vi "TestCloneAPI.vi"() -> ()   [LabVIEW 2014, in "AppModule.lvlib"]
uses:
  AppModule.lvlib
  Modules/EventPlugins/EventPluginBaseClass/TypeDefs/clEvtReportArray.ctl
  Modules/EventPlugins/EventPluginBaseClass/TypeDefs/clEvtReport.ctl
  TestInfo.ctl
  <userlib>/NIST/ModuleAdminLib/ModuleAdmin/ModuleAdmin.lvclass
  PublicAPI/Arguments/Broadcasts/clDidInit.ctl
  <userlib>/NIST/ModuleAdminLib/ModuleAdmin/ModuleAdmin.lvclass/ModuleAdmin.ctl
  PublicAPI/Arguments/Requests/clStopArgument.ctl
  PublicAPI/Arguments/Broadcasts/clStatUpdate.ctl
  PublicAPI/Arguments/Broadcasts/clErrorRpt.ctl
  <userlib>/NIST/ModuleAdminLib/ModuleAdmin/Accessors/Read CloneRegRef.vi
  <userlib>/NIST/ModuleAdminLib/CloneRegistration/CloneRegistration.lvclass
  AppPlugins/AppPluginBaseClass/AppPluginsBase.lvclass
  Modules/EventPlugins/EventPluginBaseClass/EventPluginBaseClass.lvclass
panel:
  in  "Show Panel":bool=TRUE
  in  "clEvtReportArray":T1=[{"Timestamp"=0.0, "Synx"=[568.0+0.0i, 1.190780345954324-0.33374089306165294i], "Freq"=0.0, "ROCOF"=0.0, "ID"=0}, {"Timestamp"=0.016666666666666666, "Synx"=[568.0+0.0i, 1.1810969656424384-0.32546333931377436i], "Freq"=0.0, "ROCOF"=0.0, "ID"=0}, {"Timestamp"=0.03333333333333333, "Synx"=[568.0+0.0i, 1.1693115287267182-0.31671147728228455i], "Freq"=0.0, "ROCOF"=0.0, "ID"=0}, {"Timestamp"=0.05, "Synx"=[568.0+0.0i, 1.1606529094889346-0.31107310083226175i], "Freq"=0.0, "ROCOF"=0.0, "ID"=0}, {"Timestamp"=0.06666666666666667, "Synx"=[568.0+0.0i, 1.1511600610436028-0.3062276131124402i], "Freq"=0.0, "ROCOF"=0.0, "ID"=0}, {"Timestamp"=0.08333333333333333, "Synx"=[568.0+0.0i, 1.141837461613581-0.29981509873354867i], "Freq"=0.0, "ROCOF"=0.0, "ID"=0}, {"Timestamp"=0.1, "Synx"=[568.0+0.0i, 1.132999689101532-0.29386587405402154i], "Freq"=0.0, "ROCOF"=0.0, "ID"=0}, {"Timestamp"=0.11666666666666667, "Synx"=[568.0+0.0i, 1.120988242874583-0.289722818423098i], "Freq"=0.0, "ROCOF"=0.0, "ID"=0}, {"Timestamp"=0.13333333333333333, "Synx"=[568.0+0.0i, 1.1078960385040597-0.2847668931047751i], "Freq"=0.0, "ROCOF"=0.0, "ID"=0}, {"Timestamp"=0.15, "Synx"=[568.0+0.0i, 1.096899084625727-0.27749439848438295i], "Freq"=0.0, "ROCOF"=0.0, "ID"=0}, {"Timestamp"=0.16666666666666666, "Synx"=[568.0+0.0i, 1.0850742831418392-0.27039791150864656i], "Freq"=0.0, "ROCOF"=0.0, "ID"=0}, {"Timestamp"=0.18333333333333332, "Synx"=[568.0+0.0i, 1.0713145693136845-0.2651913268468527i], "Freq"=0.0, "ROCOF"=0.0, "ID"=0}, {"Timestamp"=0.2, "Synx"=[568.0+0.0i, 1.058651026567817-0.26009080544434765i], "Freq"=0.0, "ROCOF"=0.0, "ID"=0}, {"Timestamp"=0.21666666666666667, "Synx"=[568.0+0.0i, 1.047567941555359-0.2538376451665603i], "Freq"=0.0, "ROCOF"=0.0, "ID"=0}, {"Timestamp"=0.23333333333333334, "Synx"=[568.0+0.0i, 1.0372285324721322-0.24790510395917895i], "Freq"=0.0, "ROCOF"=0.0, "ID"=0}, {"Timestamp"=0.25, "Synx"=[568.0+0.0i, 1.0281270236165359-0.24308381241327934i], "Freq"=0.0, "ROCOF"=0.0, "ID"=0}, {"Timestamp"=0.26666666666666666, "Synx"=[568.0+0.0i, 1.019518023697579-0.23787936057061518i], "Freq"=0.0, "ROCOF"=0.0, "ID"=0}, {"Timestamp"=0.2833333333333333, "Synx"=[568.0+0.0i, 1.010800255948057-0.23161401369825027i], "Freq"=0.0, "ROCOF"=0.0, "ID"=0}, {"Timestamp"=0.3, "Synx"=[568.0+0.0i, 1.003674388169744-0.22570699751690862i], "Freq"=0.0, "ROCOF"=0.0, "ID"=0}, {"Timestamp"=0.31666666666666665, "Synx"=[568.0+0.0i, 0.9986163027163525-0.2209187376418739i], "Freq"=0.0, "ROCOF"=0.0, "ID"=0}, {"Timestamp"=0.3333333333333333, "Synx"=[568.0+0.0i, 0.9938645348874-0.2162117736588246i], "Freq"=0.0, "ROCOF"=0.0, "ID"=0}, {"Timestamp"=0.35, "Synx"=[568.0+0.0i, 0.9888741952521247-0.21098043381559242i], "Freq"=0.0, "ROCOF"=0.0, "ID"=0}, {"Timestamp"=0.36666666666666664, "Synx"=[568.0+0.0i, 0.9845024487867219-0.2059636015094523i], "Freq"=0.0, "ROCOF"=0.0, "ID"=0}, {"Timestamp"=0.3833333333333333, "Synx"=[568.0+0.0i, 0.9812997021203121-0.20152897973013287i], "Freq"=0.0, "ROCOF"=0.0, "ID"=0}, {"Timestamp"=0.4, "Synx"=[568.0+0.0i, 0.9796686282331802-0.19707208766276244i], "Freq"=0.0, "ROCOF"=0.0, "ID"=0}, {"Timestamp"=0.4166666666666667, "Synx"=[568.0+0.0i, 0.9793689209737946-0.19239063538468282i], "Freq"=0.0, "ROCOF"=0.0, "ID"=0}, {"Timestamp"=0.43333333333333335, "Synx"=[568.0+0.0i, 0.9791223588762832-0.1880765496182969i], "Freq"=0.0, "ROCOF"=0.0, "ID"=0}, {"Timestamp"=0.45, "Synx"=[568.0+0.0i, 0.9784076012133255-0.1844030678057659i], "Freq"=0.0, "ROCOF"=0.0, "ID"=0}, {"Timestamp"=0.4666666666666667, "Synx"=[568.0+0.0i, 0.9780437001103851-0.18098904356917112i], "Freq"=0.0, "ROCOF"=0.0, "ID"=0}, {"Timestamp"=0.48333333333333334, "Synx"=[568.0+0.0i, 0.9785362600845192-0.17758017606549348i], "Freq"=0.0, "ROCOF"=0.0, "ID"=0}, {"Timestamp"=0.5, "Synx"=[568.0+0.0i, 0.9796244098460881-0.17433591395465478i], "Freq"=0.0, "ROCOF"=0.0, "ID"=0}, {"Timestamp"=0.5166666666666666, "Synx"=[568.0+0.0i, 0.9809907883308882-0.1714080682319968i], "Freq"=0.0, "ROCOF"=0.0, "ID"=0}, {"Timestamp"=0.5333333333333333, "Synx"=[568.0+0.0i, 0.9823274872886526-0.1687723495865902i], "Freq"=0.0, "ROCOF"=0.0, "ID"=0}, {"Timestamp"=0.55, "Synx"=[568.0+0.0i, 0.983462189784411-0.16638817596516153i], "Freq"=0.0, "ROCOF"=0.0, "ID"=0}, {"Timestamp"=0.5666666666666667, "Synx"=[568.0+0.0i, 0.9845485154103119-0.16426564040278965i], "Freq"=0.0, "ROCOF"=0.0, "ID"=0}, {"Timestamp"=0.5833333333333334, "Synx"=[568.0+0.0i, 0.985584239414064-0.16246859604208552i], "Freq"=0.0, "ROCOF"=0.0, "ID"=0}, {"Timestamp"=0.6, "Synx"=[568.0+0.0i, 0.9863346432943544-0.16105384859898314i], "Freq"=0.0, "ROCOF"=0.0, "ID"=0}, {"Timestamp"=0.6166666666666667, "Synx"=[568.0+0.0i, 0.9869274594120697-0.15990173325766183i], "Freq"=0.0, "ROCOF"=0.0, "ID"=0}, {"Timestamp"=0.6333333333333333, "Synx"=[568.0+0.0i, 0.9877478039011985-0.15881079172447463i], "Freq"=0.0, "ROCOF"=0.0, "ID"=0}, {"Timestamp"=0.65, "Synx"=[568.0+0.0i, 0.9888213981027627-0.1578654238392025i], "Freq"=0.0, "ROCOF"=0.0, "ID"=0}, {"Timestamp"=0.6666666666666666, "Synx"=[568.0+0.0i, 0.9897899903655655-0.15735170958451475i], "Freq"=0.0, "ROCOF"=0.0, "ID"=0}, {"Timestamp"=0.6833333333333333, "Synx"=[568.0+0.0i, 0.9902590603581615-0.1572358602350405i], "Freq"=0.0, "ROCOF"=0.0, "ID"=0}, {"Timestamp"=0.7, "Synx"=[568.0+0.0i, 0.9900784555069161-0.1572161214368345i], "Freq"=0.0, "ROCOF"=0.0, "ID"=0}, {"Timestamp"=0.7166666666666667, "Synx"=[568.0+0.0i, 0.9895278777753364-0.15731883208372763i], "Freq"=0.0, "ROCOF"=0.0, "ID"=0}, {"Timestamp"=0.7333333333333333, "Synx"=[568.0+0.0i, 0.989080021975212-0.15783474992005986i], "Freq"=0.0, "ROCOF"=0.0, "ID"=0}, {"Timestamp"=0.75, "Synx"=[568.0+0.0i, 0.9888954176011563-0.15867390179905863i], "Freq"=0.0, "ROCOF"=0.0, "ID"=0}, {"Timestamp"=0.7666666666666666, "Synx"=[568.0+0.0i, 0.9887907146989974-0.15947984484815012i], "Freq"=0.0, "ROCOF"=0.0, "ID"=0}, {"Timestamp"=0.7833333333333333, "Synx"=[568.0+0.0i, 0.988608996673257-0.16034377151198184i], "Freq"=0.0, "ROCOF"=0.0, "ID"=0}, {"Timestamp"=0.8, "Synx"=[568.0+0.0i, 0.9883639010187703-0.1616590571620086i], "Freq"=0.0, "ROCOF"=0.0, "ID"=0}, {"Timestamp"=0.8166666666666667, "Synx"=[568.0+0.0i, 0.9881300871093198-0.16334744819900263i], "Freq"=0.0, "ROCOF"=0.0, "ID"=0}, {"Timestamp"=0.8333333333333334, "Synx"=[568.0+0.0i, 0.987935563942819-0.16500334964923496i], "Freq"=0.0, "ROCOF"=0.0, "ID"=0}, {"Timestamp"=0.85, "Synx"=[568.0+0.0i, 0.9877272718483234-0.16667789833021487i], "Freq"=0.0, "ROCOF"=0.0, "ID"=0}, {"Timestamp"=0.8666666666666667, "Synx"=[568.0+0.0i, 0.9874788298271437-0.16872615151931622i], "Freq"=0.0, "ROCOF"=0.0, "ID"=0}, {"Timestamp"=0.8833333333333333, "Synx"=[568.0+0.0i, 0.9873308956075638-0.17104345531162607i], "Freq"=0.0, "ROCOF"=0.0, "ID"=0}, {"Timestamp"=0.9, "Synx"=[568.0+0.0i, 0.9875023373183677-0.17325359135812915i], "Freq"=0.0, "ROCOF"=0.0, "ID"=0}, {"Timestamp"=0.9166666666666666, "Synx"=[568.0+0.0i, 0.9880769375409788-0.17546082716302083i], "Freq"=0.0, "ROCOF"=0.0, "ID"=0}, {"Timestamp"=0.9333333333333333, "Synx"=[568.0+0.0i, 0.9889727901975919-0.17803061343025103i], "Freq"=0.0, "ROCOF"=0.0, "ID"=0}, {"Timestamp"=0.95, "Synx"=[568.0+0.0i, 0.9900716675954723-0.18084239270538446i], "Freq"=0.0, "ROCOF"=0.0, "ID"=0}, {"Timestamp"=0.9666666666666667, "Synx"=[568.0+0.0i, 0.9913138098801285-0.18351383569509552i], "Freq"=0.0, "ROCOF"=0.0, "ID"=0}, {"Timestamp"=0.9833333333333333, "Synx"=[568.0+0.0i, 0.9927059395134809-0.18612156281840864i], "Freq"=0.0, "ROCOF"=0.0, "ID"=0}, {"Timestamp"=1.0, "Synx"=[568.0+0.0i, 0.9942725500443967-0.1889802065654681i], "Freq"=0.0, "ROCOF"=0.0, "ID"=0}, {"Timestamp"=1.0166666666666666, "Synx"=[568.0+0.0i, 0.9960210845304401-0.1919725771479106i], "Freq"=0.0, "ROCOF"=0.0, "ID"=0}, {"Timestamp"=1.0333333333333332, "Synx"=[568.0+0.0i, 0.9979834612527839-0.19478167183195672i], "Freq"=0.0, "ROCOF"=0.0, "ID"=0}, {"Timestamp"=1.05, "Synx"=[568.0+0.0i, 1.0002484972804047-0.19751167064157604i], "Freq"=0.0, "ROCOF"=0.0, "ID"=0}, {"Timestamp"=1.0666666666666667, "Synx"=[568.0+0.0i, 1.002881503846297-0.2004414761928846i], "Freq"=0.0, "ROCOF"=0.0, "ID"=0}, {"Timestamp"=1.0833333333333333, "Synx"=[568.0+0.0i, 1.0058207005416482-0.20344096741953177i], "Freq"=0.0, "ROCOF"=0.0, "ID"=0}, {"Timestamp"=1.1, "Synx"=[568.0+0.0i, 1.0088930396474078-0.2062160694422747i], "Freq"=0.0, "ROCOF"=0.0, "ID"=0}, {"Timestamp"=1.1166666666666667, "Synx"=[568.0+0.0i, 1.0119366213904846-0.20885167018899184i], "Freq"=0.0, "ROCOF"=0.0, "ID"=0}, {"Timestamp"=1.1333333333333333, "Synx"=[568.0+0.0i, 1.0149119748644622-0.2115806058800036i], "Freq"=0.0, "ROCOF"=0.0, "ID"=0}, {"Timestamp"=1.15, "Synx"=[568.0+0.0i, 1.0179056810778668-0.21429542627327752i], "Freq"=0.0, "ROCOF"=0.0, "ID"=0}, {"Timestamp"=1.1666666666666667, "Synx"=[568.0+0.0i, 1.0210247997149353-0.21677028291320208i], "Freq"=0.0, "ROCOF"=0.0, "ID"=0}, {"Timestamp"=1.1833333333333333, "Synx"=[568.0+0.0i, 1.0242904121615224-0.21909326464360904i], "Freq"=0.0, "ROCOF"=0.0, "ID"=0}, {"Timestamp"=1.2, "Synx"=[568.0+0.0i, 1.0276294409622935-0.22144760825551188i], "Freq"=0.0, "ROCOF"=0.0, "ID"=0}, {"Timestamp"=1.2166666666666666, "Synx"=[568.0+0.0i, 1.0309366382600036-0.22372454940306044i], "Freq"=0.0, "ROCOF"=0.0, "ID"=0}, {"Timestamp"=1.2333333333333334, "Synx"=[568.0+0.0i, 1.034122599519737-0.22573253429899973i], "Freq"=0.0, "ROCOF"=0.0, "ID"=0}, {"Timestamp"=1.25, "Synx"=[568.0+0.0i, 1.0371248961434893-0.22754465011227762i], "Freq"=0.0, "ROCOF"=0.0, "ID"=0}, {"Timestamp"=1.2666666666666666, "Synx"=[568.0+0.0i, 1.0399089328448776-0.22930943033456028i], "Freq"=0.0, "ROCOF"=0.0, "ID"=0}, {"Timestamp"=1.2833333333333332, "Synx"=[568.0+0.0i, 1.0424748833879-0.23094818360098296i], "Freq"=0.0, "ROCOF"=0.0, "ID"=0}, {"Timestamp"=1.3, "Synx"=[568.0+0.0i, 1.0448588007734052-0.23232432995386262i], "Freq"=0.0, "ROCOF"=0.0, "ID"=0}, {"Timestamp"=1.3166666666666667, "Synx"=[568.0+0.0i, 1.0471046614265525-0.2334997597566502i], "Freq"=0.0, "ROCOF"=0.0, "ID"=0}, {"Timestamp"=1.3333333333333333, "Synx"=[568.0+0.0i, 1.0492147693375238-0.2345797734322047i], "Freq"=0.0, "ROCOF"=0.0, "ID"=0}, {"Timestamp"=1.35, "Synx"=[568.0+0.0i, 1.051127469782084-0.23549558631738093i], "Freq"=0.0, "ROCOF"=0.0, "ID"=0}, {"Timestamp"=1.3666666666666667, "Synx"=[568.0+0.0i, 1.0527518253261423-0.23614499855661975i], "Freq"=0.0, "ROCOF"=0.0, "ID"=0}, {"Timestamp"=1.3833333333333333, "Synx"=[568.0+0.0i, 1.0540260126145868-0.23657909568574823i], "Freq"=0.0, "ROCOF"=0.0, "ID"=0}, {"Timestamp"=1.4, "Synx"=[568.0+0.0i, 1.054945892663717-0.2368819323041705i], "Freq"=0.0, "ROCOF"=0.0, "ID"=0}, {"Timestamp"=1.4166666666666667, "Synx"=[568.0+0.0i, 1.0555482675331331-0.23701405871573272i], "Freq"=0.0, "ROCOF"=0.0, "ID"=0}, {"Timestamp"=1.4333333333333333, "Synx"=[568.0+0.0i, 1.0558754196772442-0.23691094249154757i], "Freq"=0.0, "ROCOF"=0.0, "ID"=0}, {"Timestamp"=1.45, "Synx"=[568.0+0.0i, 1.0559544563236483-0.23660818628452154i], "Freq"=0.0, "ROCOF"=0.0, "ID"=0}, {"Timestamp"=1.4666666666666666, "Synx"=[568.0+0.0i, 1.055797989100892-0.23616063145396285i], "Freq"=0.0, "ROCOF"=0.0, "ID"=0}, {"Timestamp"=1.4833333333333334, "Synx"=[568.0+0.0i, 1.055406843586187-0.23554395055091526i], "Freq"=0.0, "ROCOF"=0.0, "ID"=0}, {"Timestamp"=1.5, "Synx"=[568.0+0.0i, 1.054764636174528-0.2347207410253123i], "Freq"=0.0, "ROCOF"=0.0, "ID"=0}, {"Timestamp"=1.5166666666666666, "Synx"=[568.0+0.0i, 1.053839485044776-0.23371891599675987i], "Freq"=0.0, "ROCOF"=0.0, "ID"=0}, {"Timestamp"=1.5333333333333332, "Synx"=[568.0+0.0i, 1.052606256276664-0.23258210431801657i], "Freq"=0.0, "ROCOF"=0.0, "ID"=0}, {"Timestamp"=1.55, "Synx"=[568.0+0.0i, 1.0510755677912442-0.23130805513800712i], "Freq"=0.0, "ROCOF"=0.0, "ID"=0}, {"Timestamp"=1.5666666666666667, "Synx"=[568.0+0.0i, 1.049301705484443-0.2298801248778193i], "Freq"=0.0, "ROCOF"=0.0, "ID"=0}, {"Timestamp"=1.5833333333333333, "Synx"=[568.0+0.0i, 1.0473582415628429-0.22831163248547198i], "Freq"=0.0, "ROCOF"=0.0, "ID"=0}, {"Timestamp"=1.6, "Synx"=[568.0+0.0i, 1.045299722988945-0.2266294223502902i], "Freq"=0.0, "ROCOF"=0.0, "ID"=0}, {"Timestamp"=1.6166666666666667, "Synx"=[568.0+0.0i, 1.0431401466637653-0.22484454637484289i], "Freq"=0.0, "ROCOF"=0.0, "ID"=0}, {"Timestamp"=1.6333333333333333, "Synx"=[568.0+0.0i, 1.040861588268909-0.22295697150093405i], "Freq"=0.0, "ROCOF"=0.0, "ID"=0}, {"Timestamp"=1.65, "Synx"=[568.0+0.0i, 1.0384399620313718-0.22097421707535697i], "Freq"=0.0, "ROCOF"=0.0, "ID"=0}, {"Timestamp"=1.6666666666666667, "Synx"=[568.0+0.0i, 1.0358675042297611-0.21891745552321926i], "Freq"=0.0, "ROCOF"=0.0, "ID"=0}, {"Timestamp"=1.6833333333333333, "Synx"=[568.0+0.0i, 1.0331629251005825-0.21681001277654294i], "Freq"=0.0, "ROCOF"=0.0, "ID"=0}, {"Timestamp"=1.7, "Synx"=[568.0+0.0i, 1.0303703614372581-0.2146595394080782i], "Freq"=0.0, "ROCOF"=0.0, "ID"=0}, {"Timestamp"=1.7166666666666666, "Synx"=[568.0+0.0i, 1.0275489835542104-0.21246241961811713i], "Freq"=0.0, "ROCOF"=0.0, "ID"=0}, {"Timestamp"=1.7333333333333334, "Synx"=[568.0+0.0i, 1.0247542957426232-0.2102314718081312i], "Freq"=0.0, "ROCOF"=0.0, "ID"=0}, {"Timestamp"=1.75, "Synx"=[568.0+0.0i, 1.0220173416906368-0.20799789534335755i], "Freq"=0.0, "ROCOF"=0.0, "ID"=0}, {"Timestamp"=1.7666666666666666, "Synx"=[568.0+0.0i, 1.0193349786964445-0.2057764748395524i], "Freq"=0.0, "ROCOF"=0.0, "ID"=0}, {"Timestamp"=1.7833333333333332, "Synx"=[568.0+0.0i, 1.0166813461179105-0.20355939974713314i], "Freq"=0.0, "ROCOF"=0.0, "ID"=0}, {"Timestamp"=1.8, "Synx"=[568.0+0.0i, 1.0140349586059054-0.2013562244167269i], "Freq"=0.0, "ROCOF"=0.0, "ID"=0}, {"Timestamp"=1.8166666666666667, "Synx"=[568.0+0.0i, 1.011401946309843-0.199201567979025i], "Freq"=0.0, "ROCOF"=0.0, "ID"=0}, {"Timestamp"=1.8333333333333333, "Synx"=[568.0+0.0i, 1.0088189657709958-0.19710976685721138i], "Freq"=0.0, "ROCOF"=0.0, "ID"=0}, {"Timestamp"=1.8499999999999999, "Synx"=[568.0+0.0i, 1.0063360973300026-0.19506592883055504i], "Freq"=0.0, "ROCOF"=0.0, "ID"=0}, {"Timestamp"=1.8666666666666667, "Synx"=[568.0+0.0i, 1.0039941235484178-0.19307571606837412i], "Freq"=0.0, "ROCOF"=0.0, "ID"=0}, {"Timestamp"=1.8833333333333333, "Synx"=[568.0+0.0i, 1.0018108504340801-0.19117557136705798i], "Freq"=0.0, "ROCOF"=0.0, "ID"=0}, {"Timestamp"=1.9, "Synx"=[568.0+0.0i, 0.9997811138555077-0.1893803254456488i], "Freq"=0.0, "ROCOF"=0.0, "ID"=0}, {"Timestamp"=1.9166666666666667, "Synx"=[568.0+0.0i, 0.9978862013971358-0.18767229377489536i], "Freq"=0.0, "ROCOF"=0.0, "ID"=0}, {"Timestamp"=1.9333333333333333, "Synx"=[568.0+0.0i, 0.9961067328730887-0.1860544329617271i], "Freq"=0.0, "ROCOF"=0.0, "ID"=0}, {"Timestamp"=1.95, "Synx"=[568.0+0.0i, 0.9944347806515849-0.18456035273097823i], "Freq"=0.0, "ROCOF"=0.0, "ID"=0}, {"Timestamp"=1.9666666666666666, "Synx"=[568.0+0.0i, 0.9928809871930054-0.183200624078482i], "Freq"=0.0, "ROCOF"=0.0, "ID"=0}, {"Timestamp"=1.9833333333333334, "Synx"=[568.0+0.0i, 0.991472195404676-0.18195400575743148i], "Freq"=0.0, "ROCOF"=0.0, "ID"=0}, {"Timestamp"=2.0, "Synx"=[568.0+0.0i, 0.9902390140964307-0.18082137861780578i], "Freq"=0.0, "ROCOF"=0.0, "ID"=0}, {"Timestamp"=2.0166666666666666, "Synx"=[568.0+0.0i, 0.9891998068808097-0.17983365869239556i], "Freq"=0.0, "ROCOF"=0.0, "ID"=0}, {"Timestamp"=2.033333333333333, "Synx"=[568.0+0.0i, 0.9883513468000275-0.17899859462260528i], "Freq"=0.0, "ROCOF"=0.0, "ID"=0}, {"Timestamp"=2.05, "Synx"=[568.0+0.0i, 0.9876722603689594-0.1782935810602652i], "Freq"=0.0, "ROCOF"=0.0, "ID"=0}, {"Timestamp"=2.0666666666666664, "Synx"=[568.0+0.0i, 0.9871363571572059-0.17771691091941522i], "Freq"=0.0, "ROCOF"=0.0, "ID"=0}, {"Timestamp"=2.0833333333333335, "Synx"=[568.0+0.0i, 0.9867267773227768-0.1772936545888048i], "Freq"=0.0, "ROCOF"=0.0, "ID"=0}, {"Timestamp"=2.1, "Synx"=[568.0+0.0i, 0.9864430423534721-0.1770267626387451i], "Freq"=0.0, "ROCOF"=0.0, "ID"=0}, {"Timestamp"=2.1166666666666667, "Synx"=[568.0+0.0i, 0.986298827687823-0.17689282953983645i], "Freq"=0.0, "ROCOF"=0.0, "ID"=0}, {"Timestamp"=2.1333333333333333, "Synx"=[568.0+0.0i, 0.9863131477619512-0.1768887579439425i], "Freq"=0.0, "ROCOF"=0.0, "ID"=0}, {"Timestamp"=2.15, "Synx"=[568.0+0.0i, 0.9864994558429381-0.177034793451872i], "Freq"=0.0, "ROCOF"=0.0, "ID"=0}, {"Timestamp"=2.1666666666666665, "Synx"=[568.0+0.0i, 0.9868572194198217-0.1773304474284138i], "Freq"=0.0, "ROCOF"=0.0, "ID"=0}, {"Timestamp"=2.183333333333333, "Synx"=[568.0+0.0i, 0.9873699279289171-0.17775230993232238i], "Freq"=0.0, "ROCOF"=0.0, "ID"=0}, {"Timestamp"=2.2, "Synx"=[568.0+0.0i, 0.9880113409407102-0.17829500158520384i], "Freq"=0.0, "ROCOF"=0.0, "ID"=0}, {"Timestamp"=2.216666666666667, "Synx"=[568.0+0.0i, 0.9887574643840766-0.17897253600781066i], "Freq"=0.0, "ROCOF"=0.0, "ID"=0}, {"Timestamp"=2.2333333333333334, "Synx"=[568.0+0.0i, 0.9895975289188882-0.1797808520503357i], "Freq"=0.0, "ROCOF"=0.0, "ID"=0}, {"Timestamp"=2.25, "Synx"=[568.0+0.0i, 0.9905370349611532-0.18069754891558917i], "Freq"=0.0, "ROCOF"=0.0, "ID"=0}, {"Timestamp"=2.2666666666666666, "Synx"=[568.0+0.0i, 0.9915908737833355-0.18171619390982416i], "Freq"=0.0, "ROCOF"=0.0, "ID"=0}, {"Timestamp"=2.283333333333333, "Synx"=[568.0+0.0i, 0.9927710926045651-0.18284584848506485i], "Freq"=0.0, "ROCOF"=0.0, "ID"=0}, {"Timestamp"=2.3, "Synx"=[568.0+0.0i, 0.9940769861581061-0.18407991133459486i], "Freq"=0.0, "ROCOF"=0.0, "ID"=0}, {"Timestamp"=2.3166666666666664, "Synx"=[568.0+0.0i, 0.9954929513614348-0.18539704332928741i], "Freq"=0.0, "ROCOF"=0.0, "ID"=0}, {"Timestamp"=2.3333333333333335, "Synx"=[568.0+0.0i, 0.9969943464528188-0.1867891587045225i], "Freq"=0.0, "ROCOF"=0.0, "ID"=0}, {"Timestamp"=2.35, "Synx"=[568.0+0.0i, 0.9985573425247952-0.1882603465051167i], "Freq"=0.0, "ROCOF"=0.0, "ID"=0}, {"Timestamp"=2.3666666666666667, "Synx"=[568.0+0.0i, 1.000167483038519-0.1898022846290975i], "Freq"=0.0, "ROCOF"=0.0, "ID"=0}, {"Timestamp"=2.3833333333333333, "Synx"=[568.0+0.0i, 1.0018229554400828-0.1913957013938104i], "Freq"=0.0, "ROCOF"=0.0, "ID"=0}, {"Timestamp"=2.4, "Synx"=[568.0+0.0i, 1.0035312090473962-0.193031959160047i], "Freq"=0.0, "ROCOF"=0.0, "ID"=0}, {"Timestamp"=2.4166666666666665, "Synx"=[568.0+0.0i, 1.0053006517591185-0.19471146411512794i], "Freq"=0.0, "ROCOF"=0.0, "ID"=0}, {"Timestamp"=2.433333333333333, "Synx"=[568.0+0.0i, 1.0071317484332953-0.1964249403531514i], "Freq"=0.0, "ROCOF"=0.0, "ID"=0}, {"Timestamp"=2.45, "Synx"=[568.0+0.0i, 1.0090124582136468-0.19815504239043605i], "Freq"=0.0, "ROCOF"=0.0, "ID"=0}, {"Timestamp"=2.466666666666667, "Synx"=[568.0+0.0i, 1.0109206703555722-0.19989252092690646i], "Freq"=0.0, "ROCOF"=0.0, "ID"=0}, {"Timestamp"=2.4833333333333334, "Synx"=[568.0+0.0i, 1.0128321538239238-0.20163494496273376i], "Freq"=0.0, "ROCOF"=0.0, "ID"=0}, {"Timestamp"=2.5, "Synx"=[568.0+0.0i, 1.0147292338719154-0.20337322647478442i], "Freq"=0.0, "ROCOF"=0.0, "ID"=0}, {"Timestamp"=2.5166666666666666, "Synx"=[568.0+0.0i, 1.0166052330789968-0.20509277039788493i], "Freq"=0.0, "ROCOF"=0.0, "ID"=0}, {"Timestamp"=2.533333333333333, "Synx"=[568.0+0.0i, 1.018462594764228-0.2067846555469391i], "Freq"=0.0, "ROCOF"=0.0, "ID"=0}, {"Timestamp"=2.55, "Synx"=[568.0+0.0i, 1.0203063349318222-0.2084447732784657i], "Freq"=0.0, "ROCOF"=0.0, "ID"=0}, {"Timestamp"=2.5666666666666664, "Synx"=[568.0+0.0i, 1.0221366959972835-0.21006478864608596i], "Freq"=0.0, "ROCOF"=0.0, "ID"=0}, {"Timestamp"=2.5833333333333335, "Synx"=[568.0+0.0i, 1.0239447597183418-0.21163276568005002i], "Freq"=0.0, "ROCOF"=0.0, "ID"=0}, {"Timestamp"=2.6, "Synx"=[568.0+0.0i, 1.0257129589008291-0.21314046586550892i], "Freq"=0.0, "ROCOF"=0.0, "ID"=0}, {"Timestamp"=2.6166666666666667, "Synx"=[568.0+0.0i, 1.027420017866818-0.21458324661005146i], "Freq"=0.0, "ROCOF"=0.0, "ID"=0}, {"Timestamp"=2.6333333333333333, "Synx"=[568.0+0.0i, 1.0290477789233554-0.21595454514215445i], "Freq"=0.0, "ROCOF"=0.0, "ID"=0}, {"Timestamp"=2.65, "Synx"=[568.0+0.0i, 1.0305864073218247-0.21724562789289598i], "Freq"=0.0, "ROCOF"=0.0, "ID"=0}, {"Timestamp"=2.6666666666666665, "Synx"=[568.0+0.0i, 1.0320352004463418-0.21844964155200813i], "Freq"=0.0, "ROCOF"=0.0, "ID"=0}, {"Timestamp"=2.683333333333333, "Synx"=[568.0+0.0i, 1.033398558605959-0.21956228647542675i], "Freq"=0.0, "ROCOF"=0.0, "ID"=0}, {"Timestamp"=2.7, "Synx"=[568.0+0.0i, 1.0346794259610796-0.220579103490274i], "Freq"=0.0, "ROCOF"=0.0, "ID"=0}, {"Timestamp"=2.716666666666667, "Synx"=[568.0+0.0i, 1.0358739695934602-0.22149449595483597i], "Freq"=0.0, "ROCOF"=0.0, "ID"=0}, {"Timestamp"=2.7333333333333334, "Synx"=[568.0+0.0i, 1.0369704525709336-0.22230344771707009i], "Freq"=0.0, "ROCOF"=0.0, "ID"=0}, {"Timestamp"=2.75, "Synx"=[568.0+0.0i, 1.037952730864153-0.22300295686017155i], "Freq"=0.0, "ROCOF"=0.0, "ID"=0}, {"Timestamp"=2.7666666666666666, "Synx"=[568.0+0.0i, 1.0388062152341506-0.22359127274266685i], "Freq"=0.0, "ROCOF"=0.0, "ID"=0}, {"Timestamp"=2.783333333333333, "Synx"=[568.0+0.0i, 1.0395229873649514-0.22406610431184215i], "Freq"=0.0, "ROCOF"=0.0, "ID"=0}, {"Timestamp"=2.8, "Synx"=[568.0+0.0i, 1.0401034718302804-0.22442460907944128i], "Freq"=0.0, "ROCOF"=0.0, "ID"=0}, {"Timestamp"=2.8166666666666664, "Synx"=[568.0+0.0i, 1.0405540106953015-0.2246655131641988i], "Freq"=0.0, "ROCOF"=0.0, "ID"=0}, {"Timestamp"=2.8333333333333335, "Synx"=[568.0+0.0i, 1.040881788358684-0.22478976692268932i], "Freq"=0.0, "ROCOF"=0.0, "ID"=0}, {"Timestamp"=2.85, "Synx"=[568.0+0.0i, 1.0410898451192874-0.22479817513687864i], "Freq"=0.0, "ROCOF"=0.0, "ID"=0}, {"Timestamp"=2.8666666666666667, "Synx"=[568.0+0.0i, 1.0411748272008872-0.22469027892540053i], "Freq"=0.0, "ROCOF"=0.0, "ID"=0}, {"Timestamp"=2.8833333333333333, "Synx"=[568.0+0.0i, 1.0411286539854963-0.2244669659399703i], "Freq"=0.0, "ROCOF"=0.0, "ID"=0}, {"Timestamp"=2.9, "Synx"=[568.0+0.0i, 1.0409431383184042-0.2241319236944976i], "Freq"=0.0, "ROCOF"=0.0, "ID"=0}, {"Timestamp"=2.9166666666666665, "Synx"=[568.0+0.0i, 1.0406149486083935-0.223688776483113i], "Freq"=0.0, "ROCOF"=0.0, "ID"=0}, {"Timestamp"=2.933333333333333, "Synx"=[568.0+0.0i, 1.0401481469543568-0.22313931511734783i], "Freq"=0.0, "ROCOF"=0.0, "ID"=0}, {"Timestamp"=2.95, "Synx"=[568.0+0.0i, 1.0395529880638208-0.22248648096840987i], "Freq"=0.0, "ROCOF"=0.0, "ID"=0}, {"Timestamp"=2.966666666666667, "Synx"=[568.0+0.0i, 1.0388418160687836-0.22173628896227382i], "Freq"=0.0, "ROCOF"=0.0, "ID"=0}, {"Timestamp"=2.9833333333333334, "Synx"=[568.0+0.0i, 1.038024445035296-0.22089469991740576i], "Freq"=0.0, "ROCOF"=0.0, "ID"=0}, {"Timestamp"=3.0, "Synx"=[568.0+0.0i, 1.0371055193036594-0.21996554495909618i], "Freq"=0.0, "ROCOF"=0.0, "ID"=0}, {"Timestamp"=3.0166666666666666, "Synx"=[568.0+0.0i, 1.0360851111409897-0.21895365241069248i], "Freq"=0.0, "ROCOF"=0.0, "ID"=0}, {"Timestamp"=3.033333333333333, "Synx"=[568.0+0.0i, 1.0349620308096652-0.21786687915385072i], "Freq"=0.0, "ROCOF"=0.0, "ID"=0}, {"Timestamp"=3.05, "Synx"=[568.0+0.0i, 1.0337379556267012-0.21671286730600722i], "Freq"=0.0, "ROCOF"=0.0, "ID"=0}, {"Timestamp"=3.0666666666666664, "Synx"=[568.0+0.0i, 1.032420159355366-0.21549694207410314i], "Freq"=0.0, "ROCOF"=0.0, "ID"=0}, {"Timestamp"=3.0833333333333335, "Synx"=[568.0+0.0i, 1.0310214330160141-0.21422527222805923i], "Freq"=0.0, "ROCOF"=0.0, "ID"=0}, {"Timestamp"=3.1, "Synx"=[568.0+0.0i, 1.0295573001613536-0.21290685068428078i], "Freq"=0.0, "ROCOF"=0.0, "ID"=0}, {"Timestamp"=3.1166666666666667, "Synx"=[568.0+0.0i, 1.0280420678045863-0.21155030329001417i], "Freq"=0.0, "ROCOF"=0.0, "ID"=0}, {"Timestamp"=3.1333333333333333, "Synx"=[568.0+0.0i, 1.026485849307144-0.21016190288057138i], "Freq"=0.0, "ROCOF"=0.0, "ID"=0}, {"Timestamp"=3.15, "Synx"=[568.0+0.0i, 1.0248941098278908-0.20874858319455356i], "Freq"=0.0, "ROCOF"=0.0, "ID"=0}, {"Timestamp"=3.1666666666666665, "Synx"=[568.0+0.0i, 1.0232698513994773-0.20731971500730859i], "Freq"=0.0, "ROCOF"=0.0, "ID"=0}, {"Timestamp"=3.183333333333333, "Synx"=[568.0+0.0i, 1.0216171056391063-0.20588410095269838i], "Freq"=0.0, "ROCOF"=0.0, "ID"=0}, {"Timestamp"=3.2, "Synx"=[568.0+0.0i, 1.019943757010864-0.2044482358246055i], "Freq"=0.0, "ROCOF"=0.0, "ID"=0}, {"Timestamp"=3.216666666666667, "Synx"=[568.0+0.0i, 1.0182621888817098-0.2030191018882827i], "Freq"=0.0, "ROCOF"=0.0, "ID"=0}, {"Timestamp"=3.2333333333333334, "Synx"=[568.0+0.0i, 1.0165874904108576-0.2016056949152871i], "Freq"=0.0, "ROCOF"=0.0, "ID"=0}, {"Timestamp"=3.25, "Synx"=[568.0+0.0i, 1.0149342620899795-0.20021629454728956i], "Freq"=0.0, "ROCOF"=0.0, "ID"=0}, {"Timestamp"=3.2666666666666666, "Synx"=[568.0+0.0i, 1.0133137368991374-0.19885698972394428i], "Freq"=0.0, "ROCOF"=0.0, "ID"=0}, {"Timestamp"=3.283333333333333, "Synx"=[568.0+0.0i, 1.0117326922007803-0.19753415568661703i], "Freq"=0.0, "ROCOF"=0.0, "ID"=0}, {"Timestamp"=3.3, "Synx"=[568.0+0.0i, 1.0101946352320756-0.1962557062861227i], "Freq"=0.0, "ROCOF"=0.0, "ID"=0}, {"Timestamp"=3.3166666666666664, "Synx"=[568.0+0.0i, 1.0087025314481806-0.1950287202110056i], "Freq"=0.0, "ROCOF"=0.0, "ID"=0}, {"Timestamp"=3.3333333333333335, "Synx"=[568.0+0.0i, 1.0072615430318437-0.19385826181023505i], "Freq"=0.0, "ROCOF"=0.0, "ID"=0}, {"Timestamp"=3.35, "Synx"=[568.0+0.0i, 1.005880279054299-0.19274951304727636i], "Freq"=0.0, "ROCOF"=0.0, "ID"=0}, {"Timestamp"=3.3666666666666667, "Synx"=[568.0+0.0i, 1.0045699077788675-0.19170876632512351i], "Freq"=0.0, "ROCOF"=0.0, "ID"=0}, {"Timestamp"=3.3833333333333333, "Synx"=[568.0+0.0i, 1.003341668412867-0.19074142641550254i], "Freq"=0.0, "ROCOF"=0.0, "ID"=0}, {"Timestamp"=3.4, "Synx"=[568.0+0.0i, 1.0022041752236373-0.1898510876973532i], "Freq"=0.0, "ROCOF"=0.0, "ID"=0}, {"Timestamp"=3.4166666666666665, "Synx"=[568.0+0.0i, 1.0011619643035912-0.18904129443643466i], "Freq"=0.0, "ROCOF"=0.0, "ID"=0}, {"Timestamp"=3.433333333333333, "Synx"=[568.0+0.0i, 1.0002159963486787-0.1883163110222497i], "Freq"=0.0, "ROCOF"=0.0, "ID"=0}, {"Timestamp"=3.4499999999999997, "Synx"=[568.0+0.0i, 0.9993657447576055-0.18767952143268934i], "Freq"=0.0, "ROCOF"=0.0, "ID"=0}, {"Timestamp"=3.466666666666667, "Synx"=[568.0+0.0i, 0.9986116726251671-0.18713274128551685i], "Freq"=0.0, "ROCOF"=0.0, "ID"=0}, {"Timestamp"=3.4833333333333334, "Synx"=[568.0+0.0i, 0.9979567561916559-0.18667761728176166i], "Freq"=0.0, "ROCOF"=0.0, "ID"=0}, {"Timestamp"=3.5, "Synx"=[568.0+0.0i, 0.997406281290491-0.1863162092713793i], "Freq"=0.0, "ROCOF"=0.0, "ID"=0}, {"Timestamp"=3.5166666666666666, "Synx"=[568.0+0.0i, 0.9969660891386926-0.18604975936115342i], "Freq"=0.0, "ROCOF"=0.0, "ID"=0}, {"Timestamp"=3.533333333333333, "Synx"=[568.0+0.0i, 0.9966402670447526-0.18587818594586064i], "Freq"=0.0, "ROCOF"=0.0, "ID"=0}, {"Timestamp"=3.55, "Synx"=[568.0+0.0i, 0.9964295424714044-0.18580114488753546i], "Freq"=0.0, "ROCOF"=0.0, "ID"=0}, {"Timestamp"=3.5666666666666664, "Synx"=[568.0+0.0i, 0.9963312203782239-0.185818473874469i], "Freq"=0.0, "ROCOF"=0.0, "ID"=0}, {"Timestamp"=3.5833333333333335, "Synx"=[568.0+0.0i, 0.9963406449134696-0.18592930964841095i], "Freq"=0.0, "ROCOF"=0.0, "ID"=0}, {"Timestamp"=3.6, "Synx"=[568.0+0.0i, 0.9964533451459586-0.18613172626604754i], "Freq"=0.0, "ROCOF"=0.0, "ID"=0}, {"Timestamp"=3.6166666666666667, "Synx"=[568.0+0.0i, 0.9966666891072367-0.18642349180843512i], "Freq"=0.0, "ROCOF"=0.0, "ID"=0}, {"Timestamp"=3.6333333333333333, "Synx"=[568.0+0.0i, 0.9969801872409653-0.18680240689624547i], "Freq"=0.0, "ROCOF"=0.0, "ID"=0}, {"Timestamp"=3.65, "Synx"=[568.0+0.0i, 0.9973943537224486-0.18726571901813266i], "Freq"=0.0, "ROCOF"=0.0, "ID"=0}, {"Timestamp"=3.6666666666666665, "Synx"=[568.0+0.0i, 0.9979088128423509-0.18780986160987279i], "Freq"=0.0, "ROCOF"=0.0, "ID"=0}, {"Timestamp"=3.683333333333333, "Synx"=[568.0+0.0i, 0.9985207085784669-0.18843095232817975i], "Freq"=0.0, "ROCOF"=0.0, "ID"=0}, {"Timestamp"=3.6999999999999997, "Synx"=[568.0+0.0i, 0.9992242646278583-0.1891250659624096i], "Freq"=0.0, "ROCOF"=0.0, "ID"=0}, {"Timestamp"=3.716666666666667, "Synx"=[568.0+0.0i, 1.0000116934124799-0.18988790243732154i], "Freq"=0.0, "ROCOF"=0.0, "ID"=0}, {"Timestamp"=3.7333333333333334, "Synx"=[568.0+0.0i, 1.0008749290986005-0.19071459337633773i], "Freq"=0.0, "ROCOF"=0.0, "ID"=0}, {"Timestamp"=3.75, "Synx"=[568.0+0.0i, 1.0018072441448587-0.1915999838259529i], "Freq"=0.0, "ROCOF"=0.0, "ID"=0}, {"Timestamp"=3.7666666666666666, "Synx"=[568.0+0.0i, 1.0028039076667605-0.1925388599034244i], "Freq"=0.0, "ROCOF"=0.0, "ID"=0}, {"Timestamp"=3.783333333333333, "Synx"=[568.0+0.0i, 1.003861587242621-0.19352581616107542i], "Freq"=0.0, "ROCOF"=0.0, "ID"=0}, {"Timestamp"=3.8, "Synx"=[568.0+0.0i, 1.0049768802801915-0.19455510318750538i], "Freq"=0.0, "ROCOF"=0.0, "ID"=0}, {"Timestamp"=3.8166666666666664, "Synx"=[568.0+0.0i, 1.0061448146314809-0.19562074210389557i], "Freq"=0.0, "ROCOF"=0.0, "ID"=0}, {"Timestamp"=3.8333333333333335, "Synx"=[568.0+0.0i, 1.007358142859756-0.1967167298637634i], "Freq"=0.0, "ROCOF"=0.0, "ID"=0}, {"Timestamp"=3.85, "Synx"=[568.0+0.0i, 1.00860779497357-0.19783705895208065i], "Freq"=0.0, "ROCOF"=0.0, "ID"=0}, {"Timestamp"=3.8666666666666667, "Synx"=[568.0+0.0i, 1.0098842169175037-0.19897558468448356i], "Freq"=0.0, "ROCOF"=0.0, "ID"=0}, {"Timestamp"=3.8833333333333333, "Synx"=[568.0+0.0i, 1.011178858818969-0.20012601108108485i], "Freq"=0.0, "ROCOF"=0.0, "ID"=0}, {"Timestamp"=3.9, "Synx"=[568.0+0.0i, 1.0124850289927154-0.20128208217084906i], "Freq"=0.0, "ROCOF"=0.0, "ID"=0}, {"Timestamp"=3.9166666666666665, "Synx"=[568.0+0.0i, 1.0137977026271638-0.2024377084594979i], "Freq"=0.0, "ROCOF"=0.0, "ID"=0}, {"Timestamp"=3.933333333333333, "Synx"=[568.0+0.0i, 1.0151124491394243-0.20358684260411145i], "Freq"=0.0, "ROCOF"=0.0, "ID"=0}, {"Timestamp"=3.9499999999999997, "Synx"=[568.0+0.0i, 1.0164241049721945-0.20472337713513603i], "Freq"=0.0, "ROCOF"=0.0, "ID"=0}, {"Timestamp"=3.966666666666667, "Synx"=[568.0+0.0i, 1.0177259288041245-0.205841329585249i], "Freq"=0.0, "ROCOF"=0.0, "ID"=0}, {"Timestamp"=3.9833333333333334, "Synx"=[568.0+0.0i, 1.0190096893671852-0.2069350364625256i], "Freq"=0.0, "ROCOF"=0.0, "ID"=0}, {"Timestamp"=4.0, "Synx"=[568.0+0.0i, 1.0202666194943035-0.20799902742409807i], "Freq"=0.0, "ROCOF"=0.0, "ID"=0}, {"Timestamp"=4.016666666666667, "Synx"=[568.0+0.0i, 1.021488707710869-0.20902786387932934i], "Freq"=0.0, "ROCOF"=0.0, "ID"=0}, {"Timestamp"=4.033333333333333, "Synx"=[568.0+0.0i, 1.0226696370562114-0.21001631794052444i], "Freq"=0.0, "ROCOF"=0.0, "ID"=0}, {"Timestamp"=4.05, "Synx"=[568.0+0.0i, 1.023804896655799-0.2109596019987795i], "Freq"=0.0, "ROCOF"=0.0, "ID"=0}, {"Timestamp"=4.066666666666666, "Synx"=[568.0+0.0i, 1.024891054591562-0.21185323977060794i], "Freq"=0.0, "ROCOF"=0.0, "ID"=0}, {"Timestamp"=4.083333333333333, "Synx"=[568.0+0.0i, 1.0259246310194525-0.2126928728625221i], "Freq"=0.0, "ROCOF"=0.0, "ID"=0}, {"Timestamp"=4.1, "Synx"=[568.0+0.0i, 1.0269012057368159-0.21347443219995235i], "Freq"=0.0, "ROCOF"=0.0, "ID"=0}, {"Timestamp"=4.116666666666666, "Synx"=[568.0+0.0i, 1.027815240693725-0.21419437644345046i], "Freq"=0.0, "ROCOF"=0.0, "ID"=0}, {"Timestamp"=4.133333333333333, "Synx"=[568.0+0.0i, 1.0286606936923244-0.21484955774275472i], "Freq"=0.0, "ROCOF"=0.0, "ID"=0}, {"Timestamp"=4.15, "Synx"=[568.0+0.0i, 1.0294320724175916-0.2154370143219451i], "Freq"=0.0, "ROCOF"=0.0, "ID"=0}, {"Timestamp"=4.166666666666667, "Synx"=[568.0+0.0i, 1.0301253567065425-0.21595413077151254i], "Freq"=0.0, "ROCOF"=0.0, "ID"=0}, {"Timestamp"=4.183333333333334, "Synx"=[568.0+0.0i, 1.030738310204174-0.21639886717395307i], "Freq"=0.0, "ROCOF"=0.0, "ID"=0}, {"Timestamp"=4.2, "Synx"=[568.0+0.0i, 1.0312700473211396-0.2167696224841078i], "Freq"=0.0, "ROCOF"=0.0, "ID"=0}, {"Timestamp"=4.216666666666667, "Synx"=[568.0+0.0i, 1.0317201238690874-0.21706502780097908i], "Freq"=0.0, "ROCOF"=0.0, "ID"=0}, {"Timestamp"=4.233333333333333, "Synx"=[568.0+0.0i, 1.0320876628160311-0.21728409112310762i], "Freq"=0.0, "ROCOF"=0.0, "ID"=0}, {"Timestamp"=4.25, "Synx"=[568.0+0.0i, 1.0323709862346906-0.2174264030755045i], "Freq"=0.0, "ROCOF"=0.0, "ID"=0}, {"Timestamp"=4.266666666666667, "Synx"=[568.0+0.0i, 1.0325679330832016-0.2174919997093849i], "Freq"=0.0, "ROCOF"=0.0, "ID"=0}, {"Timestamp"=4.283333333333333, "Synx"=[568.0+0.0i, 1.0326766662033717-0.2174811655541134i], "Freq"=0.0, "ROCOF"=0.0, "ID"=0}, {"Timestamp"=4.3, "Synx"=[568.0+0.0i, 1.032696516494469-0.21739455963329707i], "Freq"=0.0, "ROCOF"=0.0, "ID"=0}, {"Timestamp"=4.316666666666666, "Synx"=[568.0+0.0i, 1.032628409902785-0.21723339101287625i], "Freq"=0.0, "ROCOF"=0.0, "ID"=0}, {"Timestamp"=4.333333333333333, "Synx"=[568.0+0.0i, 1.0324746641150886-0.2169992851653377i], "Freq"=0.0, "ROCOF"=0.0, "ID"=0}, {"Timestamp"=4.35, "Synx"=[568.0+0.0i, 1.0322382867936144-0.21669410280284668i], "Freq"=0.0, "ROCOF"=0.0, "ID"=0}, {"Timestamp"=4.366666666666666, "Synx"=[568.0+0.0i, 1.0319221668510608-0.21632004405306698i], "Freq"=0.0, "ROCOF"=0.0, "ID"=0}, {"Timestamp"=4.383333333333333, "Synx"=[568.0+0.0i, 1.0315285897927267-0.21587978996140247i], "Freq"=0.0, "ROCOF"=0.0, "ID"=0}, {"Timestamp"=4.4, "Synx"=[568.0+0.0i, 1.031059315962401-0.21537637559723927i], "Freq"=0.0, "ROCOF"=0.0, "ID"=0}, {"Timestamp"=4.416666666666667, "Synx"=[568.0+0.0i, 1.0305161487793255-0.21481302811973807i], "Freq"=0.0, "ROCOF"=0.0, "ID"=0}, {"Timestamp"=4.433333333333334, "Synx"=[568.0+0.0i, 1.0299016598775008-0.21419324858157454i], "Freq"=0.0, "ROCOF"=0.0, "ID"=0}, {"Timestamp"=4.45, "Synx"=[568.0+0.0i, 1.029219666363022-0.2135209204612558i], "Freq"=0.0, "ROCOF"=0.0, "ID"=0}, {"Timestamp"=4.466666666666667, "Synx"=[568.0+0.0i, 1.0284752032510356-0.212800193207802i], "Freq"=0.0, "ROCOF"=0.0, "ID"=0}, {"Timestamp"=4.483333333333333, "Synx"=[568.0+0.0i, 1.0276740139011808-0.21203534086222092i], "Freq"=0.0, "ROCOF"=0.0, "ID"=0}, {"Timestamp"=4.5, "Synx"=[568.0+0.0i, 1.0268218377851666-0.21123082152003722i], "Freq"=0.0, "ROCOF"=0.0, "ID"=0}, {"Timestamp"=4.516666666666667, "Synx"=[568.0+0.0i, 1.0259238714142305-0.21039135567697023i], "Freq"=0.0, "ROCOF"=0.0, "ID"=0}, {"Timestamp"=4.533333333333333, "Synx"=[568.0+0.0i, 1.0249846693590385-0.20952182320869708i], "Freq"=0.0, "ROCOF"=0.0, "ID"=0}, {"Timestamp"=4.55, "Synx"=[568.0+0.0i, 1.0240085048941572-0.20862714319845982i], "Freq"=0.0, "ROCOF"=0.0, "ID"=0}, {"Timestamp"=4.566666666666666, "Synx"=[568.0+0.0i, 1.0229999623391008-0.20771231341341118i], "Freq"=0.0, "ROCOF"=0.0, "ID"=0}, {"Timestamp"=4.583333333333333, "Synx"=[568.0+0.0i, 1.0219644181800682-0.20678246365890895i], "Freq"=0.0, "ROCOF"=0.0, "ID"=0}, {"Timestamp"=4.6, "Synx"=[568.0+0.0i, 1.0209081414341832-0.20584276862808254i], "Freq"=0.0, "ROCOF"=0.0, "ID"=0}, {"Timestamp"=4.616666666666666, "Synx"=[568.0+0.0i, 1.019837958287597-0.2048983482948202i], "Freq"=0.0, "ROCOF"=0.0, "ID"=0}, {"Timestamp"=4.633333333333333, "Synx"=[568.0+0.0i, 1.0187606612577174-0.2039542901482685i], "Freq"=0.0, "ROCOF"=0.0, "ID"=0}, {"Timestamp"=4.65, "Synx"=[568.0+0.0i, 1.0176824724470745-0.20301568323249433i], "Freq"=0.0, "ROCOF"=0.0, "ID"=0}, {"Timestamp"=4.666666666666667, "Synx"=[568.0+0.0i, 1.0166088290059523-0.20208754869715048i], "Freq"=0.0, "ROCOF"=0.0, "ID"=0}, {"Timestamp"=4.683333333333334, "Synx"=[568.0+0.0i, 1.0155445757016979-0.20117476017908312i], "Freq"=0.0, "ROCOF"=0.0, "ID"=0}, {"Timestamp"=4.7, "Synx"=[568.0+0.0i, 1.0144944282605235-0.2002820527688007i], "Freq"=0.0, "ROCOF"=0.0, "ID"=0}, {"Timestamp"=4.716666666666667, "Synx"=[568.0+0.0i, 1.0134634319864066-0.1994140437502579i], "Freq"=0.0, "ROCOF"=0.0, "ID"=0}, {"Timestamp"=4.733333333333333, "Synx"=[568.0+0.0i, 1.0124571543964993-0.19857518159877913i], "Freq"=0.0, "ROCOF"=0.0, "ID"=0}, {"Timestamp"=4.75, "Synx"=[568.0+0.0i, 1.011481504371806-0.19776968495819794i], "Freq"=0.0, "ROCOF"=0.0, "ID"=0}, {"Timestamp"=4.766666666666667, "Synx"=[568.0+0.0i, 1.0105422754123117-0.19700154216335072i], "Freq"=0.0, "ROCOF"=0.0, "ID"=0}, {"Timestamp"=4.783333333333333, "Synx"=[568.0+0.0i, 1.0096446549572584-0.19627452418880523i], "Freq"=0.0, "ROCOF"=0.0, "ID"=0}, {"Timestamp"=4.8, "Synx"=[568.0+0.0i, 1.0087929506207438-0.19559215223284185i], "Freq"=0.0, "ROCOF"=0.0, "ID"=0}, {"Timestamp"=4.816666666666666, "Synx"=[568.0+0.0i, 1.0079906585542548-0.19495765400981588i], "Freq"=0.0, "ROCOF"=0.0, "ID"=0}, {"Timestamp"=4.833333333333333, "Synx"=[568.0+0.0i, 1.0072408118301963-0.19437395771311453i], "Freq"=0.0, "ROCOF"=0.0, "ID"=0}, {"Timestamp"=4.85, "Synx"=[568.0+0.0i, 1.006546400456679-0.19384370174687732i], "Freq"=0.0, "ROCOF"=0.0, "ID"=0}, {"Timestamp"=4.866666666666666, "Synx"=[568.0+0.0i, 1.005910625874371-0.1933692198843506i], "Freq"=0.0, "ROCOF"=0.0, "ID"=0}, {"Timestamp"=4.883333333333333, "Synx"=[568.0+0.0i, 1.0053368521044037-0.19295251302975772i], "Freq"=0.0, "ROCOF"=0.0, "ID"=0}, {"Timestamp"=4.9, "Synx"=[568.0+0.0i, 1.004828284781337-0.19259524087171695i], "Freq"=0.0, "ROCOF"=0.0, "ID"=0}, {"Timestamp"=4.916666666666667, "Synx"=[568.0+0.0i, 1.0043875548199743-0.1922987319555496i], "Freq"=0.0, "ROCOF"=0.0, "ID"=0}, {"Timestamp"=4.933333333333334, "Synx"=[568.0+0.0i, 1.0040164284605368-0.19206398487620052i], "Freq"=0.0, "ROCOF"=0.0, "ID"=0}, {"Timestamp"=4.95, "Synx"=[568.0+0.0i, 1.003715789864982-0.1918916536401944i], "Freq"=0.0, "ROCOF"=0.0, "ID"=0}, {"Timestamp"=4.966666666666667, "Synx"=[568.0+0.0i, 1.0034858916720504-0.19178203958029608i], "Freq"=0.0, "ROCOF"=0.0, "ID"=0}, {"Timestamp"=4.983333333333333, "Synx"=[568.0+0.0i, 1.0033267267960733-0.19173510396979637i], "Freq"=0.0, "ROCOF"=0.0, "ID"=0}, {"Timestamp"=5.0, "Synx"=[568.0+0.0i, 1.0032383170353087-0.1917504828516047i], "Freq"=0.0, "ROCOF"=0.0, "ID"=0}, {"Timestamp"=5.016666666666667, "Synx"=[568.0+0.0i, 1.0032207681445935-0.19182748378399625i], "Freq"=0.0, "ROCOF"=0.0, "ID"=0}, {"Timestamp"=5.033333333333333, "Synx"=[568.0+0.0i, 1.0032740733264955-0.19196507978054253i], "Freq"=0.0, "ROCOF"=0.0, "ID"=0}, {"Timestamp"=5.05, "Synx"=[568.0+0.0i, 1.0033977835652619-0.19216192565092038i], "Freq"=0.0, "ROCOF"=0.0, "ID"=0}, {"Timestamp"=5.066666666666666, "Synx"=[568.0+0.0i, 1.003590730686606-0.19241638377355708i], "Freq"=0.0, "ROCOF"=0.0, "ID"=0}, {"Timestamp"=5.083333333333333, "Synx"=[568.0+0.0i, 1.0038509542236131-0.19272652994260053i], "Freq"=0.0, "ROCOF"=0.0, "ID"=0}, {"Timestamp"=5.1, "Synx"=[568.0+0.0i, 1.004175868899983-0.19309015022434953i], "Freq"=0.0, "ROCOF"=0.0, "ID"=0}, {"Timestamp"=5.116666666666666, "Synx"=[568.0+0.0i, 1.0045625801768623-0.19350476106002978i], "Freq"=0.0, "ROCOF"=0.0, "ID"=0}, {"Timestamp"=5.133333333333333, "Synx"=[568.0+0.0i, 1.0050081806979294-0.19396764290124094i], "Freq"=0.0, "ROCOF"=0.0, "ID"=0}, {"Timestamp"=5.15, "Synx"=[568.0+0.0i, 1.0055098783389436-0.19447585277475907i], "Freq"=0.0, "ROCOF"=0.0, "ID"=0}, {"Timestamp"=5.166666666666667, "Synx"=[568.0+0.0i, 1.0060649036030218-0.19502622427673633i], "Freq"=0.0, "ROCOF"=0.0, "ID"=0}, {"Timestamp"=5.183333333333334, "Synx"=[568.0+0.0i, 1.0066702651055675-0.19561539078837775i], "Freq"=0.0, "ROCOF"=0.0, "ID"=0}, {"Timestamp"=5.2, "Synx"=[568.0+0.0i, 1.0073225010639546-0.19623982390795303i], "Freq"=0.0, "ROCOF"=0.0, "ID"=0}, {"Timestamp"=5.216666666666667, "Synx"=[568.0+0.0i, 1.0080175713529735-0.1968958503668058i], "Freq"=0.0, "ROCOF"=0.0, "ID"=0}, {"Timestamp"=5.233333333333333, "Synx"=[568.0+0.0i, 1.008750954000322-0.19757965469950775i], "Freq"=0.0, "ROCOF"=0.0, "ID"=0}, {"Timestamp"=5.25, "Synx"=[568.0+0.0i, 1.009517898369839-0.19828730426648097i], "Freq"=0.0, "ROCOF"=0.0, "ID"=0}, {"Timestamp"=5.266666666666667, "Synx"=[568.0+0.0i, 1.0103137057438232-0.19901478947683637i], "Freq"=0.0, "ROCOF"=0.0, "ID"=0}, {"Timestamp"=5.283333333333333, "Synx"=[568.0+0.0i, 1.0111338989628946-0.19975804281680093i], "Freq"=0.0, "ROCOF"=0.0, "ID"=0}, {"Timestamp"=5.3, "Synx"=[568.0+0.0i, 1.011974208068996-0.20051294335999878i], "Freq"=0.0, "ROCOF"=0.0, "ID"=0}, {"Timestamp"=5.316666666666666, "Synx"=[568.0+0.0i, 1.0128304005333102-0.20127534203383415i], "Freq"=0.0, "ROCOF"=0.0, "ID"=0}, {"Timestamp"=5.333333333333333, "Synx"=[568.0+0.0i, 1.0136980667561373-0.20204110090717126i], "Freq"=0.0, "ROCOF"=0.0, "ID"=0}, {"Timestamp"=5.35, "Synx"=[568.0+0.0i, 1.0145724909533393-0.2028061122437551i], "Freq"=0.0, "ROCOF"=0.0, "ID"=0}, {"Timestamp"=5.366666666666666, "Synx"=[568.0+0.0i, 1.0154486864516232-0.20356630367786796i], "Freq"=0.0, "ROCOF"=0.0, "ID"=0}, {"Timestamp"=5.383333333333333, "Synx"=[568.0+0.0i, 1.0163215830353902-0.20431766200395626i], "Freq"=0.0, "ROCOF"=0.0, "ID"=0}, {"Timestamp"=5.4, "Synx"=[568.0+0.0i, 1.017186272897865-0.20505626917260925i], "Freq"=0.0, "ROCOF"=0.0, "ID"=0}, {"Timestamp"=5.416666666666667, "Synx"=[568.0+0.0i, 1.0180381939513956-0.20577831957778667i], "Freq"=0.0, "ROCOF"=0.0, "ID"=0}, {"Timestamp"=5.433333333333334, "Synx"=[568.0+0.0i, 1.0188731674461204-0.2064801246645199i], "Freq"=0.0, "ROCOF"=0.0, "ID"=0}, {"Timestamp"=5.45, "Synx"=[568.0+0.0i, 1.019687287870982-0.20715813362910207i], "Freq"=0.0, "ROCOF"=0.0, "ID"=0}, {"Timestamp"=5.466666666666667, "Synx"=[568.0+0.0i, 1.0204767418285008-0.20780896421385514i], "Freq"=0.0, "ROCOF"=0.0, "ID"=0}, {"Timestamp"=5.483333333333333, "Synx"=[568.0+0.0i, 1.0212376669482748-0.20842941671823828i], "Freq"=0.0, "ROCOF"=0.0, "ID"=0}, {"Timestamp"=5.5, "Synx"=[568.0+0.0i, 1.0219661353679779-0.2090164768094309i], "Freq"=0.0, "ROCOF"=0.0, "ID"=0}, {"Timestamp"=5.516666666666667, "Synx"=[568.0+0.0i, 1.022658275575987-0.20956733173869277i], "Freq"=0.0, "ROCOF"=0.0, "ID"=0}, {"Timestamp"=5.533333333333333, "Synx"=[568.0+0.0i, 1.0233104711490006-0.21007939455433494i], "Freq"=0.0, "ROCOF"=0.0, "ID"=0}, {"Timestamp"=5.55, "Synx"=[568.0+0.0i, 1.0239195355971182-0.21055031373185776i], "Freq"=0.0, "ROCOF"=0.0, "ID"=0}, {"Timestamp"=5.566666666666666, "Synx"=[568.0+0.0i, 1.024482778726415-0.21097797316322878i], "Freq"=0.0, "ROCOF"=0.0, "ID"=0}, {"Timestamp"=5.583333333333333, "Synx"=[568.0+0.0i, 1.0249979407111536-0.2113605028517062i], "Freq"=0.0, "ROCOF"=0.0, "ID"=0}, {"Timestamp"=5.6, "Synx"=[568.0+0.0i, 1.0254630410800945-0.2116962956869903i], "Freq"=0.0, "ROCOF"=0.0, "ID"=0}, {"Timestamp"=5.616666666666666, "Synx"=[568.0+0.0i, 1.0258762326320552-0.2119840119736437i], "Freq"=0.0, "ROCOF"=0.0, "ID"=0}, {"Timestamp"=5.633333333333333, "Synx"=[568.0+0.0i, 1.0262357431408762-0.2122225758454484i], "Freq"=0.0, "ROCOF"=0.0, "ID"=0}, {"Timestamp"=5.65, "Synx"=[568.0+0.0i, 1.0265399364697667-0.21241117984147273i], "Freq"=0.0, "ROCOF"=0.0, "ID"=0}, {"Timestamp"=5.666666666666667, "Synx"=[568.0+0.0i, 1.0267874586350758-0.21254929396092387i], "Freq"=0.0, "ROCOF"=0.0, "ID"=0}, {"Timestamp"=5.683333333333334, "Synx"=[568.0+0.0i, 1.0269773894303111-0.2126366648296583i], "Freq"=0.0, "ROCOF"=0.0, "ID"=0}, {"Timestamp"=5.7, "Synx"=[568.0+0.0i, 1.0271093196300742-0.21267330816440977i], "Freq"=0.0, "ROCOF"=0.0, "ID"=0}, {"Timestamp"=5.716666666666667, "Synx"=[568.0+0.0i, 1.0271833160397073-0.21265950710959472i], "Freq"=0.0, "ROCOF"=0.0, "ID"=0}, {"Timestamp"=5.733333333333333, "Synx"=[568.0+0.0i, 1.0271997973722957-0.21259581381102438i], "Freq"=0.0, "ROCOF"=0.0, "ID"=0}, {"Timestamp"=5.75, "Synx"=[568.0+0.0i, 1.0271593898685838-0.21248304339029167i], "Freq"=0.0, "ROCOF"=0.0, "ID"=0}, {"Timestamp"=5.766666666666667, "Synx"=[568.0+0.0i, 1.0270628387511458-0.2123222624951767i], "Freq"=0.0, "ROCOF"=0.0, "ID"=0}, {"Timestamp"=5.783333333333333, "Synx"=[568.0+0.0i, 1.0269110177718923-0.2121147817793899i], "Freq"=0.0, "ROCOF"=0.0, "ID"=0}, {"Timestamp"=5.8, "Synx"=[568.0+0.0i, 1.0267050240640663-0.21186215074935488i], "Freq"=0.0, "ROCOF"=0.0, "ID"=0}, {"Timestamp"=5.816666666666666, "Synx"=[568.0+0.0i, 1.0264462995872217-0.2115661471530367i], "Freq"=0.0, "ROCOF"=0.0, "ID"=0}, {"Timestamp"=5.833333333333333, "Synx"=[568.0+0.0i, 1.0261367078722872-0.2112287620722902i], "Freq"=0.0, "ROCOF"=0.0, "ID"=0}, {"Timestamp"=5.85, "Synx"=[568.0+0.0i, 1.0257785209086585-0.2108521873778944i], "Freq"=0.0, "ROCOF"=0.0, "ID"=0}, {"Timestamp"=5.866666666666666, "Synx"=[568.0+0.0i, 1.0253743202915657-0.21043880502271173i], "Freq"=0.0, "ROCOF"=0.0, "ID"=0}, {"Timestamp"=5.883333333333333, "Synx"=[568.0+0.0i, 1.0249268618384257-0.20999117282257618i], "Freq"=0.0, "ROCOF"=0.0, "ID"=0}, {"Timestamp"=5.9, "Synx"=[568.0+0.0i, 1.0244389698227974-0.20951200693322497i], "Freq"=0.0, "ROCOF"=0.0, "ID"=0}, {"Timestamp"=5.916666666666667, "Synx"=[568.0+0.0i, 1.0239135078543238-0.20900416551069814i], "Freq"=0.0, "ROCOF"=0.0, "ID"=0}, {"Timestamp"=5.933333333333334, "Synx"=[568.0+0.0i, 1.0233534299718436-0.20847063396657708i], "Freq"=0.0, "ROCOF"=0.0, "ID"=0}, {"Timestamp"=5.95, "Synx"=[568.0+0.0i, 1.0227618719809528-0.2079145084163386i], "Freq"=0.0, "ROCOF"=0.0, "ID"=0}, {"Timestamp"=5.966666666666667, "Synx"=[568.0+0.0i, 1.022142222765238-0.20733897668418672i], "Freq"=0.0, "ROCOF"=0.0, "ID"=0}, {"Timestamp"=5.983333333333333, "Synx"=[568.0+0.0i, 1.021498128147648-0.20674729967071157i], "Freq"=0.0, "ROCOF"=0.0, "ID"=0}, {"Timestamp"=6.0, "Synx"=[568.0+0.0i, 1.0208334176405367-0.20614279429029359i], "Freq"=0.0, "ROCOF"=0.0, "ID"=0}, {"Timestamp"=6.016666666666667, "Synx"=[568.0+0.0i, 1.0201519858666082-0.20552881604780754i], "Freq"=0.0, "ROCOF"=0.0, "ID"=0}, {"Timestamp"=6.033333333333333, "Synx"=[568.0+0.0i, 1.0194576832234792-0.20490873991398156i], "Freq"=0.0, "ROCOF"=0.0, "ID"=0}, {"Timestamp"=6.05, "Synx"=[568.0+0.0i, 1.0187542630660906-0.20428594105425504i], "Freq"=0.0, "ROCOF"=0.0, "ID"=0}, {"Timestamp"=6.066666666666666, "Synx"=[568.0+0.0i, 1.0180454004335766-0.20366377724140172i], "Freq"=0.0, "ROCOF"=0.0, "ID"=0}, {"Timestamp"=6.083333333333333, "Synx"=[568.0+0.0i, 1.0173347584360033-0.20304557207577323i], "Freq"=0.0, "ROCOF"=0.0, "ID"=0}, {"Timestamp"=6.1, "Synx"=[568.0+0.0i, 1.0166260539450658-0.2024345971290324i], "Freq"=0.0, "ROCOF"=0.0, "ID"=0}, {"Timestamp"=6.116666666666666, "Synx"=[568.0+0.0i, 1.0159230767086482-0.20183405367997492i], "Freq"=0.0, "ROCOF"=0.0, "ID"=0}, {"Timestamp"=6.133333333333333, "Synx"=[568.0+0.0i, 1.0152296430001035-0.20124705631630044i], "Freq"=0.0, "ROCOF"=0.0, "ID"=0}, {"Timestamp"=6.15, "Synx"=[568.0+0.0i, 1.014549500963457-0.20067661823495747i], "Freq"=0.0, "ROCOF"=0.0, "ID"=0}, {"Timestamp"=6.166666666666667, "Synx"=[568.0+0.0i, 1.0138862302545553-0.20012563597621974i], "Freq"=0.0, "ROCOF"=0.0, "ID"=0}, {"Timestamp"=6.183333333333334, "Synx"=[568.0+0.0i, 1.0132431802218138-0.19959687366545237i], "Freq"=0.0, "ROCOF"=0.0, "ID"=0}, {"Timestamp"=6.2, "Synx"=[568.0+0.0i, 1.0126234688123772-0.1990929493019679i], "Freq"=0.0, "ROCOF"=0.0, "ID"=0}, {"Timestamp"=6.216666666666667, "Synx"=[568.0+0.0i, 1.0120300314064534-0.19861632336292911i], "Freq"=0.0, "ROCOF"=0.0, "ID"=0}, {"Timestamp"=6.233333333333333, "Synx"=[568.0+0.0i, 1.0114656829748736-0.1981692872344395i], "Freq"=0.0, "ROCOF"=0.0, "ID"=0}, {"Timestamp"=6.25, "Synx"=[568.0+0.0i, 1.0109331518407374-0.197753951176059i], "Freq"=0.0, "ROCOF"=0.0, "ID"=0}, {"Timestamp"=6.266666666666667, "Synx"=[568.0+0.0i, 1.0104350607923511-0.19737223446232027i], "Freq"=0.0, "ROCOF"=0.0, "ID"=0}, {"Timestamp"=6.283333333333333, "Synx"=[568.0+0.0i, 1.0099738610631097-0.19702585819835639i], "Freq"=0.0, "ROCOF"=0.0, "ID"=0}, {"Timestamp"=6.3, "Synx"=[568.0+0.0i, 1.009551750320851-0.19671633823888654i], "Freq"=0.0, "ROCOF"=0.0, "ID"=0}, {"Timestamp"=6.316666666666666, "Synx"=[568.0+0.0i, 1.0091706137414975-0.19644497771432234i], "Freq"=0.0, "ROCOF"=0.0, "ID"=0}, {"Timestamp"=6.333333333333333, "Synx"=[568.0+0.0i, 1.0088320139546334-0.19621286177352854i], "Freq"=0.0, "ROCOF"=0.0, "ID"=0}, {"Timestamp"=6.35, "Synx"=[568.0+0.0i, 1.0085372291212298-0.19602085512474196i], "Freq"=0.0, "ROCOF"=0.0, "ID"=0}, {"Timestamp"=6.366666666666666, "Synx"=[568.0+0.0i, 1.0082873133758927-0.1958695998416328i], "Freq"=0.0, "ROCOF"=0.0, "ID"=0}, {"Timestamp"=6.383333333333333, "Synx"=[568.0+0.0i, 1.0080831436699635-0.19575951285176574i], "Freq"=0.0, "ROCOF"=0.0, "ID"=0}, {"Timestamp"=6.4, "Synx"=[568.0+0.0i, 1.0079254265332382-0.19569078557318276i], "Freq"=0.0, "ROCOF"=0.0, "ID"=0}, {"Timestamp"=6.416666666666667, "Synx"=[568.0+0.0i, 1.0078146615445531-0.19566338627014904i], "Freq"=0.0, "ROCOF"=0.0, "ID"=0}, {"Timestamp"=6.433333333333334, "Synx"=[568.0+0.0i, 1.0077510823377387-0.19567706272792604i], "Freq"=0.0, "ROCOF"=0.0, "ID"=0}, {"Timestamp"=6.45, "Synx"=[568.0+0.0i, 1.007734607867396-0.19573134465210343i], "Freq"=0.0, "ROCOF"=0.0, "ID"=0}, {"Timestamp"=6.466666666666667, "Synx"=[568.0+0.0i, 1.0077648305431648-0.19582554803494076i], "Freq"=0.0, "ROCOF"=0.0, "ID"=0}, {"Timestamp"=6.483333333333333, "Synx"=[568.0+0.0i, 1.007841047719826-0.19595878199615868i], "Freq"=0.0, "ROCOF"=0.0, "ID"=0}, {"Timestamp"=6.5, "Synx"=[568.0+0.0i, 1.0079623202454662-0.19612995590227128i], "Freq"=0.0, "ROCOF"=0.0, "ID"=0}, {"Timestamp"=6.516666666666667, "Synx"=[568.0+0.0i, 1.0081275286239941-0.19633778620261616i], "Freq"=0.0, "ROCOF"=0.0, "ID"=0}, {"Timestamp"=6.533333333333333, "Synx"=[568.0+0.0i, 1.008335400480432-0.19658080495036076i], "Freq"=0.0, "ROCOF"=0.0, "ID"=0}, {"Timestamp"=6.55, "Synx"=[568.0+0.0i, 1.0085845000801428-0.19685737042886595i], "Freq"=0.0, "ROCOF"=0.0, "ID"=0}, {"Timestamp"=6.566666666666666, "Synx"=[568.0+0.0i, 1.0088731919381742-0.19716567793859616i], "Freq"=0.0, "ROCOF"=0.0, "ID"=0}, {"Timestamp"=6.583333333333333, "Synx"=[568.0+0.0i, 1.0091996044918439-0.19750377023750895i], "Freq"=0.0, "ROCOF"=0.0, "ID"=0}, {"Timestamp"=6.6, "Synx"=[568.0+0.0i, 1.0095616192366983-0.19786954930479192i], "Freq"=0.0, "ROCOF"=0.0, "ID"=0}, {"Timestamp"=6.616666666666666, "Synx"=[568.0+0.0i, 1.0099568965423726-0.19826078975988917i], "Freq"=0.0, "ROCOF"=0.0, "ID"=0}, {"Timestamp"=6.633333333333333, "Synx"=[568.0+0.0i, 1.0103829297191271-0.19867515226897692i], "Freq"=0.0, "ROCOF"=0.0, "ID"=0}, {"Timestamp"=6.6499999999999995, "Synx"=[568.0+0.0i, 1.0108371045363154-0.19911019649379813i], "Freq"=0.0, "ROCOF"=0.0, "ID"=0}, {"Timestamp"=6.666666666666667, "Synx"=[568.0+0.0i, 1.0113167397747398-0.19956339495147388i], "Freq"=0.0, "ROCOF"=0.0, "ID"=0}, {"Timestamp"=6.683333333333334, "Synx"=[568.0+0.0i, 1.0118190958684263-0.200032148040241i], "Freq"=0.0, "ROCOF"=0.0, "ID"=0}, {"Timestamp"=6.7, "Synx"=[568.0+0.0i, 1.0123413565780426-0.20051379884758816i], "Freq"=0.0, "ROCOF"=0.0, "ID"=0}, {"Timestamp"=6.716666666666667, "Synx"=[568.0+0.0i, 1.0128806030991186-0.20100564735605836i], "Freq"=0.0, "ROCOF"=0.0, "ID"=0}, {"Timestamp"=6.733333333333333, "Synx"=[568.0+0.0i, 1.0134338034419772-0.2015049651288832i], "Freq"=0.0, "ROCOF"=0.0, "ID"=0}, {"Timestamp"=6.75, "Synx"=[568.0+0.0i, 1.0139978309401765-0.20200901067223118i], "Freq"=0.0, "ROCOF"=0.0, "ID"=0}, {"Timestamp"=6.766666666666667, "Synx"=[568.0+0.0i, 1.0145695096662446-0.20251504436753046i], "Freq"=0.0, "ROCOF"=0.0, "ID"=0}, {"Timestamp"=6.783333333333333, "Synx"=[568.0+0.0i, 1.0151456702554698-0.20302034264290236i], "Freq"=0.0, "ROCOF"=0.0, "ID"=0}, {"Timestamp"=6.8, "Synx"=[568.0+0.0i, 1.0157231947302792-0.20352221220606537i], "Freq"=0.0, "ROCOF"=0.0, "ID"=0}, {"Timestamp"=6.816666666666666, "Synx"=[568.0+0.0i, 1.016299035623175-0.20401800449800253i], "Freq"=0.0, "ROCOF"=0.0, "ID"=0}, {"Timestamp"=6.833333333333333, "Synx"=[568.0+0.0i, 1.0168702089504078-0.20450512951948177i], "Freq"=0.0, "ROCOF"=0.0, "ID"=0}, {"Timestamp"=6.85, "Synx"=[568.0+0.0i, 1.0174337744527369-0.2049810687452471i], "Freq"=0.0, "ROCOF"=0.0, "ID"=0}, {"Timestamp"=6.866666666666666, "Synx"=[568.0+0.0i, 1.0179868225893536-0.20544338772306536i], "Freq"=0.0, "ROCOF"=0.0, "ID"=0}, {"Timestamp"=6.883333333333333, "Synx"=[568.0+0.0i, 1.0185264831182472-0.20588974849898417i], "Freq"=0.0, "ROCOF"=0.0, "ID"=0}, {"Timestamp"=6.8999999999999995, "Synx"=[568.0+0.0i, 1.019049957652842-0.20631792125343554i], "Freq"=0.0, "ROCOF"=0.0, "ID"=0}, {"Timestamp"=6.916666666666667, "Synx"=[568.0+0.0i, 1.0195545653330853-0.20672579490079968i], "Freq"=0.0, "ROCOF"=0.0, "ID"=0}, {"Timestamp"=6.933333333333334, "Synx"=[568.0+0.0i, 1.0200377838183203-0.20711138706245194i], "Freq"=0.0, "ROCOF"=0.0, "ID"=0}, {"Timestamp"=6.95, "Synx"=[568.0+0.0i, 1.0204972706526574-0.20747285355282002i], "Freq"=0.0, "ROCOF"=0.0, "ID"=0}, {"Timestamp"=6.966666666666667, "Synx"=[568.0+0.0i, 1.0209308607508083-0.20780849696516712i], "Freq"=0.0, "ROCOF"=0.0, "ID"=0}, {"Timestamp"=6.983333333333333, "Synx"=[568.0+0.0i, 1.0213365482576342-0.2081167741410059i], "Freq"=0.0, "ROCOF"=0.0, "ID"=0}, {"Timestamp"=7.0, "Synx"=[568.0+0.0i, 1.0217124685822259-0.20839630278447058i], "Freq"=0.0, "ROCOF"=0.0, "ID"=0}, {"Timestamp"=7.016666666666667, "Synx"=[568.0+0.0i, 1.0220568951629048-0.2086458673709673i], "Freq"=0.0, "ROCOF"=0.0, "ID"=0}, {"Timestamp"=7.033333333333333, "Synx"=[568.0+0.0i, 1.0223682565126408-0.20886442410634623i], "Freq"=0.0, "ROCOF"=0.0, "ID"=0}, {"Timestamp"=7.05, "Synx"=[568.0+0.0i, 1.0226451674678076-0.20905110474672664i], "Freq"=0.0, "ROCOF"=0.0, "ID"=0}, {"Timestamp"=7.066666666666666, "Synx"=[568.0+0.0i, 1.0228864606512666-0.20920521942769854i], "Freq"=0.0, "ROCOF"=0.0, "ID"=0}, {"Timestamp"=7.083333333333333, "Synx"=[568.0+0.0i, 1.023091204049602-0.20932625866889984i], "Freq"=0.0, "ROCOF"=0.0, "ID"=0}, {"Timestamp"=7.1, "Synx"=[568.0+0.0i, 1.0232586980367784-0.20941389444740505i], "Freq"=0.0, "ROCOF"=0.0, "ID"=0}, {"Timestamp"=7.116666666666666, "Synx"=[568.0+0.0i, 1.0233884558677107-0.2094679801728417i], "Freq"=0.0, "ROCOF"=0.0, "ID"=0}, {"Timestamp"=7.133333333333333, "Synx"=[568.0+0.0i, 1.0234801797616884-0.20948854963237526i], "Freq"=0.0, "ROCOF"=0.0, "ID"=0}, {"Timestamp"=7.1499999999999995, "Synx"=[568.0+0.0i, 1.0235337459725793-0.20947581509052987i], "Freq"=0.0, "ROCOF"=0.0, "ID"=0}, {"Timestamp"=7.166666666666667, "Synx"=[568.0+0.0i, 1.0235492062993437-0.20943016454356364i], "Freq"=0.0, "ROCOF"=0.0, "ID"=0}, {"Timestamp"=7.183333333333334, "Synx"=[568.0+0.0i, 1.0235268038072345-0.20935215798166698i], "Freq"=0.0, "ROCOF"=0.0, "ID"=0}, {"Timestamp"=7.2, "Synx"=[568.0+0.0i, 1.0234669924469897-0.20924252267332918i], "Freq"=0.0, "ROCOF"=0.0, "ID"=0}, {"Timestamp"=7.216666666666667, "Synx"=[568.0+0.0i, 1.0233704480406158-0.20910214767424257i], "Freq"=0.0, "ROCOF"=0.0, "ID"=0}, {"Timestamp"=7.233333333333333, "Synx"=[568.0+0.0i, 1.023238062698138-0.2089320776384665i], "Freq"=0.0, "ROCOF"=0.0, "ID"=0}, {"Timestamp"=7.25, "Synx"=[568.0+0.0i, 1.0230709234030493-0.2087335058036809i], "Freq"=0.0, "ROCOF"=0.0, "ID"=0}, {"Timestamp"=7.266666666666667, "Synx"=[568.0+0.0i, 1.0228702834475891-0.2085077661321164i], "Freq"=0.0, "ROCOF"=0.0, "ID"=0}, {"Timestamp"=7.283333333333333, "Synx"=[568.0+0.0i, 1.0226375383925943-0.20825632482218i], "Freq"=0.0, "ROCOF"=0.0, "ID"=0}, {"Timestamp"=7.3, "Synx"=[568.0+0.0i, 1.0223742148731905-0.20798077132126996i], "Freq"=0.0, "ROCOF"=0.0, "ID"=0}, {"Timestamp"=7.316666666666666, "Synx"=[568.0+0.0i, 1.022081972928589-0.207682808728459i], "Freq"=0.0, "ROCOF"=0.0, "ID"=0}, {"Timestamp"=7.333333333333333, "Synx"=[568.0+0.0i, 1.0217626148709067-0.2073642435512425i], "Freq"=0.0, "ROCOF"=0.0, "ID"=0}, {"Timestamp"=7.35, "Synx"=[568.0+0.0i, 1.02141809012921-0.20702697503714948i], "Freq"=0.0, "ROCOF"=0.0, "ID"=0}, {"Timestamp"=7.366666666666666, "Synx"=[568.0+0.0i, 1.021050487760791-0.20667298424169578i], "Freq"=0.0, "ROCOF"=0.0, "ID"=0}, {"Timestamp"=7.383333333333333, "Synx"=[568.0+0.0i, 1.020662014966747-0.20630432273626415i], "Freq"=0.0, "ROCOF"=0.0, "ID"=0}, {"Timestamp"=7.3999999999999995, "Synx"=[568.0+0.0i, 1.020254967247349-0.20592310091279858i], "Freq"=0.0, "ROCOF"=0.0, "ID"=0}, {"Timestamp"=7.416666666666667, "Synx"=[568.0+0.0i, 1.0198316998517845-0.20553147610372663i], "Freq"=0.0, "ROCOF"=0.0, "ID"=0}, {"Timestamp"=7.433333333333334, "Synx"=[568.0+0.0i, 1.0193946089004187-0.20513164069125295i], "Freq"=0.0, "ROCOF"=0.0, "ID"=0}, {"Timestamp"=7.45, "Synx"=[568.0+0.0i, 1.0189461248868128-0.20472581012215707i], "Freq"=0.0, "ROCOF"=0.0, "ID"=0}, {"Timestamp"=7.466666666666667, "Synx"=[568.0+0.0i, 1.0184887144176185-0.20431621078332038i], "Freq"=0.0, "ROCOF"=0.0, "ID"=0}, {"Timestamp"=7.483333333333333, "Synx"=[568.0+0.0i, 1.0180248817361954-0.20390506794556904i], "Freq"=0.0, "ROCOF"=0.0, "ID"=0}, {"Timestamp"=7.5, "Synx"=[568.0+0.0i, 1.0175571620047195-0.20349459394780237i], "Freq"=0.0, "ROCOF"=0.0, "ID"=0}, {"Timestamp"=7.516666666666667, "Synx"=[568.0+0.0i, 1.017088103065574-0.2030869765473051i], "Freq"=0.0, "ROCOF"=0.0, "ID"=0}, {"Timestamp"=7.533333333333333, "Synx"=[568.0+0.0i, 1.0166202387479188-0.20268436739192922i], "Freq"=0.0, "ROCOF"=0.0, "ID"=0}, {"Timestamp"=7.55, "Synx"=[568.0+0.0i, 1.0161560612667675-0.20228887080294777i], "Freq"=0.0, "ROCOF"=0.0, "ID"=0}, {"Timestamp"=7.566666666666666, "Synx"=[568.0+0.0i, 1.0156980005563139-0.20190253302690087i], "Freq"=0.0, "ROCOF"=0.0, "ID"=0}, {"Timestamp"=7.583333333333333, "Synx"=[568.0+0.0i, 1.0152484144997211-0.2015273318891014i], "Freq"=0.0, "ROCOF"=0.0, "ID"=0}, {"Timestamp"=7.6, "Synx"=[568.0+0.0i, 1.014809588210829-0.20116516680468788i], "Freq"=0.0, "ROCOF"=0.0, "ID"=0}, {"Timestamp"=7.616666666666666, "Synx"=[568.0+0.0i, 1.0143837359753984-0.20081784931051289i], "Freq"=0.0, "ROCOF"=0.0, "ID"=0}, {"Timestamp"=7.633333333333333, "Synx"=[568.0+0.0i, 1.013972998552009-0.20048709425429811i], "Freq"=0.0, "ROCOF"=0.0, "ID"=0}, {"Timestamp"=7.6499999999999995, "Synx"=[568.0+0.0i, 1.01357943160046-0.20017451157753166i], "Freq"=0.0, "ROCOF"=0.0, "ID"=0}, {"Timestamp"=7.666666666666667, "Synx"=[568.0+0.0i, 1.0132049862415702-0.19988159864654345i], "Freq"=0.0, "ROCOF"=0.0, "ID"=0}, {"Timestamp"=7.683333333333334, "Synx"=[568.0+0.0i, 1.0128514872628045-0.1996097332645629i], "Freq"=0.0, "ROCOF"=0.0, "ID"=0}, {"Timestamp"=7.7, "Synx"=[568.0+0.0i, 1.0125206158823876-0.19936016747410815i], "Freq"=0.0, "ROCOF"=0.0, "ID"=0}, {"Timestamp"=7.716666666666667, "Synx"=[568.0+0.0i, 1.0122139016473668-0.19913402208743883i], "Freq"=0.0, "ROCOF"=0.0, "ID"=0}, {"Timestamp"=7.733333333333333, "Synx"=[568.0+0.0i, 1.0119327233705095-0.19893228189599085i], "Freq"=0.0, "ROCOF"=0.0, "ID"=0}, {"Timestamp"=7.75, "Synx"=[568.0+0.0i, 1.0116783146004862-0.19875579165825424i], "Freq"=0.0, "ROCOF"=0.0, "ID"=0}, {"Timestamp"=7.766666666666667, "Synx"=[568.0+0.0i, 1.0114517673173715-0.1986052529459761i], "Freq"=0.0, "ROCOF"=0.0, "ID"=0}, {"Timestamp"=7.783333333333333, "Synx"=[568.0+0.0i, 1.0112540292065386-0.19848122178579666i], "Freq"=0.0, "ROCOF"=0.0, "ID"=0}, {"Timestamp"=7.8, "Synx"=[568.0+0.0i, 1.0110858939548601-0.1983841070419642i], "Freq"=0.0, "ROCOF"=0.0, "ID"=0}, {"Timestamp"=7.816666666666666, "Synx"=[568.0+0.0i, 1.010947988241655-0.1983141696056435i], "Freq"=0.0, "ROCOF"=0.0, "ID"=0}, {"Timestamp"=7.833333333333333, "Synx"=[568.0+0.0i, 1.0108407611912793-0.19827152244136126i], "Freq"=0.0, "ROCOF"=0.0, "ID"=0}, {"Timestamp"=7.85, "Synx"=[568.0+0.0i, 1.0107644809782967-0.1982561314261176i], "Freq"=0.0, "ROCOF"=0.0, "ID"=0}, {"Timestamp"=7.866666666666666, "Synx"=[568.0+0.0i, 1.010719239733225-0.19826781692063403i], "Freq"=0.0, "ROCOF"=0.0, "ID"=0}, {"Timestamp"=7.883333333333333, "Synx"=[568.0+0.0i, 1.010704963882031-0.19830625610587616i], "Freq"=0.0, "ROCOF"=0.0, "ID"=0}, {"Timestamp"=7.8999999999999995, "Synx"=[568.0+0.0i, 1.0107214247319627-0.19837098610831314i], "Freq"=0.0, "ROCOF"=0.0, "ID"=0}, {"Timestamp"=7.916666666666667, "Synx"=[568.0+0.0i, 1.01076824466018-0.19846140784791413i], "Freq"=0.0, "ROCOF"=0.0, "ID"=0}, {"Timestamp"=7.933333333333334, "Synx"=[568.0+0.0i, 1.0108448972590907-0.19857679054237942i], "Freq"=0.0, "ROCOF"=0.0, "ID"=0}, {"Timestamp"=7.95, "Synx"=[568.0+0.0i, 1.0109507035357803-0.1987162768718856i], "Freq"=0.0, "ROCOF"=0.0, "ID"=0}, {"Timestamp"=7.966666666666667, "Synx"=[568.0+0.0i, 1.0110848287156868-0.1988788888046705i], "Freq"=0.0, "ROCOF"=0.0, "ID"=0}, {"Timestamp"=7.983333333333333, "Synx"=[568.0+0.0i, 1.0112462841005263-0.19906353401696963i], "Freq"=0.0, "ROCOF"=0.0, "ID"=0}, {"Timestamp"=8.0, "Synx"=[568.0+0.0i, 1.0114339359336288-0.1992690128361973i], "Freq"=0.0, "ROCOF"=0.0, "ID"=0}, {"Timestamp"=8.016666666666666, "Synx"=[568.0+0.0i, 1.0116465197652438-0.19949402568783034i], "Freq"=0.0, "ROCOF"=0.0, "ID"=0}, {"Timestamp"=8.033333333333333, "Synx"=[568.0+0.0i, 1.0118826562762875-0.19973718102831783i], "Freq"=0.0, "ROCOF"=0.0, "ID"=0}, {"Timestamp"=8.05, "Synx"=[568.0+0.0i, 1.012140864228289-0.1999970036989048i], "Freq"=0.0, "ROCOF"=0.0, "ID"=0}, {"Timestamp"=8.066666666666666, "Synx"=[568.0+0.0i, 1.0124195682221575-0.20027194362704048i], "Freq"=0.0, "ROCOF"=0.0, "ID"=0}, {"Timestamp"=8.083333333333334, "Synx"=[568.0+0.0i, 1.012717102094335-0.2005603848380858i], "Freq"=0.0, "ROCOF"=0.0, "ID"=0}, {"Timestamp"=8.1, "Synx"=[568.0+0.0i, 1.0130317113243317-0.20086065474744683i], "Freq"=0.0, "ROCOF"=0.0, "ID"=0}, {"Timestamp"=8.116666666666667, "Synx"=[568.0+0.0i, 1.0133615584335007-0.20117103367185635i], "Freq"=0.0, "ROCOF"=0.0, "ID"=0}, {"Timestamp"=8.133333333333333, "Synx"=[568.0+0.0i, 1.013704733775563-0.20148976448734604i], "Freq"=0.0, "ROCOF"=0.0, "ID"=0}, {"Timestamp"=8.15, "Synx"=[568.0+0.0i, 1.0140592712891323-0.20181506238545513i], "Freq"=0.0, "ROCOF"=0.0, "ID"=0}, {"Timestamp"=8.166666666666666, "Synx"=[568.0+0.0i, 1.014423166267186-0.20214512469156729i], "Freq"=0.0, "ROCOF"=0.0, "ID"=0}, {"Timestamp"=8.183333333333334, "Synx"=[568.0+0.0i, 1.0147943913312643-0.20247814069066247i], "Freq"=0.0, "ROCOF"=0.0, "ID"=0}, {"Timestamp"=8.2, "Synx"=[568.0+0.0i, 1.0151709079756268-0.20281230139236425i], "Freq"=0.0, "ROCOF"=0.0, "ID"=0}, {"Timestamp"=8.216666666666667, "Synx"=[568.0+0.0i, 1.015550673554509-0.20314580918218614i], "Freq"=0.0, "ROCOF"=0.0, "ID"=0}, {"Timestamp"=8.233333333333333, "Synx"=[568.0+0.0i, 1.0159316460270795-0.2034768873223038i], "Freq"=0.0, "ROCOF"=0.0, "ID"=0}, {"Timestamp"=8.25, "Synx"=[568.0+0.0i, 1.0163117898458331-0.2038037892563836i], "Freq"=0.0, "ROCOF"=0.0, "ID"=0}, {"Timestamp"=8.266666666666666, "Synx"=[568.0+0.0i, 1.0166890855581956-0.20412480765812124i], "Freq"=0.0, "ROCOF"=0.0, "ID"=0}, {"Timestamp"=8.283333333333333, "Synx"=[568.0+0.0i, 1.0170615435028938-0.20443828317175644i], "Freq"=0.0, "ROCOF"=0.0, "ID"=0}, {"Timestamp"=8.3, "Synx"=[568.0+0.0i, 1.0174272196506038-0.2047426128122968i], "Freq"=0.0, "ROCOF"=0.0, "ID"=0}, {"Timestamp"=8.316666666666666, "Synx"=[568.0+0.0i, 1.0177842304177191-0.20503625799155614i], "Freq"=0.0, "ROCOF"=0.0, "ID"=0}, {"Timestamp"=8.333333333333334, "Synx"=[568.0+0.0i, 1.0181307637817918-0.20531775212047945i], "Freq"=0.0, "ROCOF"=0.0, "ID"=0}, {"Timestamp"=8.35, "Synx"=[568.0+0.0i, 1.018465085910454-0.2055857077424728i], "Freq"=0.0, "ROCOF"=0.0, "ID"=0}, {"Timestamp"=8.366666666666667, "Synx"=[568.0+0.0i, 1.0187855447189345-0.2058388231738601i], "Freq"=0.0, "ROCOF"=0.0, "ID"=0}, {"Timestamp"=8.383333333333333, "Synx"=[568.0+0.0i, 1.019090573103524-0.20607588863086115i], "Freq"=0.0, "ROCOF"=0.0, "ID"=0}, {"Timestamp"=8.4, "Synx"=[568.0+0.0i, 1.019378694383652-0.20629579180673233i], "Freq"=0.0, "ROCOF"=0.0, "ID"=0}, {"Timestamp"=8.416666666666666, "Synx"=[568.0+0.0i, 1.01964853090361-0.20649752286413114i], "Freq"=0.0, "ROCOF"=0.0, "ID"=0}, {"Timestamp"=8.433333333333334, "Synx"=[568.0+0.0i, 1.0198988147009003-0.20668017882999964i], "Freq"=0.0, "ROCOF"=0.0, "ID"=0}, {"Timestamp"=8.45, "Synx"=[568.0+0.0i, 1.0201283977566826-0.20684296738657357i], "Freq"=0.0, "ROCOF"=0.0, "ID"=0}, {"Timestamp"=8.466666666666667, "Synx"=[568.0+0.0i, 1.0203362593249343-0.20698521003675543i], "Freq"=0.0, "ROCOF"=0.0, "ID"=0}, {"Timestamp"=8.483333333333333, "Synx"=[568.0+0.0i, 1.02052150914648-0.207106344621788i], "Freq"=0.0, "ROCOF"=0.0, "ID"=0}, {"Timestamp"=8.5, "Synx"=[568.0+0.0i, 1.0206833872385628-0.20720592719118436i], "Freq"=0.0, "ROCOF"=0.0, "ID"=0}, {"Timestamp"=8.516666666666666, "Synx"=[568.0+0.0i, 1.0208212623797948-0.20728363323274385i], "Freq"=0.0, "ROCOF"=0.0, "ID"=0}, {"Timestamp"=8.533333333333333, "Synx"=[568.0+0.0i, 1.0209346316397985-0.20733925825587965i], "Freq"=0.0, "ROCOF"=0.0, "ID"=0}, {"Timestamp"=8.55, "Synx"=[568.0+0.0i, 1.0210231222611275-0.20737271772017277i], "Freq"=0.0, "ROCOF"=0.0, "ID"=0}, {"Timestamp"=8.566666666666666, "Synx"=[568.0+0.0i, 1.0210864954999193-0.20738404632197424i], "Freq"=0.0, "ROCOF"=0.0, "ID"=0}, {"Timestamp"=8.583333333333334, "Synx"=[568.0+0.0i, 1.0211246506110274-0.20737339666017518i], "Freq"=0.0, "ROCOF"=0.0, "ID"=0}, {"Timestamp"=8.6, "Synx"=[568.0+0.0i, 1.021137626774111-0.2073410372886778i], "Freq"=0.0, "ROCOF"=0.0, "ID"=0}, {"Timestamp"=8.616666666666667, "Synx"=[568.0+0.0i, 1.0211256015675345-0.20728735016119504i], "Freq"=0.0, "ROCOF"=0.0, "ID"=0}, {"Timestamp"=8.633333333333333, "Synx"=[568.0+0.0i, 1.0210888861259049-0.20721282749306885i], "Freq"=0.0, "ROCOF"=0.0, "ID"=0}, {"Timestamp"=8.65, "Synx"=[568.0+0.0i, 1.0210279185186613-0.20711806807269165i], "Freq"=0.0, "ROCOF"=0.0, "ID"=0}, {"Timestamp"=8.666666666666666, "Synx"=[568.0+0.0i, 1.0209432574181612-0.2070037730426832i], "Freq"=0.0, "ROCOF"=0.0, "ID"=0}, {"Timestamp"=8.683333333333334, "Synx"=[568.0+0.0i, 1.020835577539377-0.2068707411686739i], "Freq"=0.0, "ROCOF"=0.0, "ID"=0}, {"Timestamp"=8.7, "Synx"=[568.0+0.0i, 1.020705666991065-0.206719863630215i], "Freq"=0.0, "ROCOF"=0.0, "ID"=0}, {"Timestamp"=8.716666666666667, "Synx"=[568.0+0.0i, 1.020554425331224-0.20655211837527773i], "Freq"=0.0, "ROCOF"=0.0, "ID"=0}, {"Timestamp"=8.733333333333333, "Synx"=[568.0+0.0i, 1.0203828604906844-0.2063685640685565i], "Freq"=0.0, "ROCOF"=0.0, "ID"=0}, {"Timestamp"=8.75, "Synx"=[568.0+0.0i, 1.0201920831264428-0.20617033366115417i], "Freq"=0.0, "ROCOF"=0.0, "ID"=0}, {"Timestamp"=8.766666666666666, "Synx"=[568.0+0.0i, 1.0199832981371952-0.20595862762315761i], "Freq"=0.0, "ROCOF"=0.0, "ID"=0}, {"Timestamp"=8.783333333333333, "Synx"=[568.0+0.0i, 1.0197577943601832-0.20573470688626555i], "Freq"=0.0, "ROCOF"=0.0, "ID"=0}, {"Timestamp"=8.8, "Synx"=[568.0+0.0i, 1.019516934178525-0.20549988553354165i], "Freq"=0.0, "ROCOF"=0.0, "ID"=0}, {"Timestamp"=8.816666666666666, "Synx"=[568.0+0.0i, 1.0192621445461676-0.2052555232703736i], "Freq"=0.0, "ROCOF"=0.0, "ID"=0}, {"Timestamp"=8.833333333333334, "Synx"=[568.0+0.0i, 1.0189949099413644-0.20500301772175314i], "Freq"=0.0, "ROCOF"=0.0, "ID"=0}, {"Timestamp"=8.85, "Synx"=[568.0+0.0i, 1.018716766554919-0.20474379660521663i], "Freq"=0.0, "ROCOF"=0.0, "ID"=0}, {"Timestamp"=8.866666666666667, "Synx"=[568.0+0.0i, 1.0184292962603032-0.204479309819776i], "Freq"=0.0, "ROCOF"=0.0, "ID"=0}, {"Timestamp"=8.883333333333333, "Synx"=[568.0+0.0i, 1.0181341189877298-0.2042110214877893i], "Freq"=0.0, "ROCOF"=0.0, "ID"=0}, {"Timestamp"=8.9, "Synx"=[568.0+0.0i, 1.0178328829592713-0.2039404019948775i], "Freq"=0.0, "ROCOF"=0.0, "ID"=0}, {"Timestamp"=8.916666666666666, "Synx"=[568.0+0.0i, 1.0175272533592112-0.20366892007579404i], "Freq"=0.0, "ROCOF"=0.0, "ID"=0}, {"Timestamp"=8.933333333333334, "Synx"=[568.0+0.0i, 1.0172189008034054-0.20339803498613584i], "Freq"=0.0, "ROCOF"=0.0, "ID"=0}, {"Timestamp"=8.95, "Synx"=[568.0+0.0i, 1.016909491024198-0.20312918879599876i], "Freq"=0.0, "ROCOF"=0.0, "ID"=0}, {"Timestamp"=8.966666666666667, "Synx"=[568.0+0.0i, 1.016600676505049-0.20286379884713482i], "Freq"=0.0, "ROCOF"=0.0, "ID"=0}, {"Timestamp"=8.983333333333333, "Synx"=[568.0+0.0i, 1.0162940897765511-0.20260325041666344i], "Freq"=0.0, "ROCOF"=0.0, "ID"=0}, {"Timestamp"=9.0, "Synx"=[568.0+0.0i, 1.015991337283729-0.20234888962328718i], "Freq"=0.0, "ROCOF"=0.0, "ID"=0}, {"Timestamp"=9.016666666666666, "Synx"=[568.0+0.0i, 1.0156939925729245-0.20210201660779387i], "Freq"=0.0, "ROCOF"=0.0, "ID"=0}, {"Timestamp"=9.033333333333333, "Synx"=[568.0+0.0i, 1.0154035880846957-0.20186387902268127i], "Freq"=0.0, "ROCOF"=0.0, "ID"=0}, {"Timestamp"=9.05, "Synx"=[568.0+0.0i, 1.0151216057593657-0.20163566586613765i], "Freq"=0.0, "ROCOF"=0.0, "ID"=0}, {"Timestamp"=9.066666666666666, "Synx"=[568.0+0.0i, 1.0148494674548942-0.20141850168936906i], "Freq"=0.0, "ROCOF"=0.0, "ID"=0}, {"Timestamp"=9.083333333333334, "Synx"=[568.0+0.0i, 1.0145885264222283-0.2012134412017939i], "Freq"=0.0, "ROCOF"=0.0, "ID"=0}, {"Timestamp"=9.1, "Synx"=[568.0+0.0i, 1.0143400606710726-0.20102146429967513i], "Freq"=0.0, "ROCOF"=0.0, "ID"=0}, {"Timestamp"=9.116666666666667, "Synx"=[568.0+0.0i, 1.0141052682354403-0.2008434715433234i], "Freq"=0.0, "ROCOF"=0.0, "ID"=0}, {"Timestamp"=9.133333333333333, "Synx"=[568.0+0.0i, 1.0138852635698352-0.200680280102595i], "Freq"=0.0, "ROCOF"=0.0, "ID"=0}, {"Timestamp"=9.15, "Synx"=[568.0+0.0i, 1.0136810739868836-0.2005326201857739i], "Freq"=0.0, "ROCOF"=0.0, "ID"=0}, {"Timestamp"=9.166666666666666, "Synx"=[568.0+0.0i, 1.013493635336783-0.20040113196642248i], "Freq"=0.0, "ROCOF"=0.0, "ID"=0}, {"Timestamp"=9.183333333333334, "Synx"=[568.0+0.0i, 1.0133237868464617-0.2002863630218128i], "Freq"=0.0, "ROCOF"=0.0, "ID"=0}, {"Timestamp"=9.2, "Synx"=[568.0+0.0i, 1.0131722657786504-0.20018876629197416i], "Freq"=0.0, "ROCOF"=0.0, "ID"=0}, {"Timestamp"=9.216666666666667, "Synx"=[568.0+0.0i, 1.013039702938111-0.20010869856377628i], "Freq"=0.0, "ROCOF"=0.0, "ID"=0}, {"Timestamp"=9.233333333333333, "Synx"=[568.0+0.0i, 1.012926619861295-0.20004641948287832i], "Freq"=0.0, "ROCOF"=0.0, "ID"=0}, {"Timestamp"=9.25, "Synx"=[568.0+0.0i, 1.012833427900122-0.20000209109517242i], "Freq"=0.0, "ROCOF"=0.0, "ID"=0}, {"Timestamp"=9.266666666666666, "Synx"=[568.0+0.0i, 1.0127604287014074-0.19997577791562793i], "Freq"=0.0, "ROCOF"=0.0, "ID"=0}, {"Timestamp"=9.283333333333333, "Synx"=[568.0+0.0i, 1.0127078151720255-0.19996744751804965i], "Freq"=0.0, "ROCOF"=0.0, "ID"=0}, {"Timestamp"=9.3, "Synx"=[568.0+0.0i, 1.012675672112599-0.19997697163705486i], "Freq"=0.0, "ROCOF"=0.0, "ID"=0}, {"Timestamp"=9.316666666666666, "Synx"=[568.0+0.0i, 1.0126639762272944-0.200004127772423i], "Freq"=0.0, "ROCOF"=0.0, "ID"=0}, {"Timestamp"=9.333333333333334, "Synx"=[568.0+0.0i, 1.0126725958739637-0.20004860128314353i], "Freq"=0.0, "ROCOF"=0.0, "ID"=0}, {"Timestamp"=9.35, "Synx"=[568.0+0.0i, 1.0127012913487936-0.20010998795451782i], "Freq"=0.0, "ROCOF"=0.0, "ID"=0}, {"Timestamp"=9.366666666666667, "Synx"=[568.0+0.0i, 1.012749716480419-0.2001877970192683i], "Freq"=0.0, "ROCOF"=0.0, "ID"=0}, {"Timestamp"=9.383333333333333, "Synx"=[568.0+0.0i, 1.0128174218672625-0.2002814546127559i], "Freq"=0.0, "ROCOF"=0.0, "ID"=0}, {"Timestamp"=9.4, "Synx"=[568.0+0.0i, 1.0129038594806954-0.200390307640494i], "Freq"=0.0, "ROCOF"=0.0, "ID"=0}, {"Timestamp"=9.416666666666666, "Synx"=[568.0+0.0i, 1.0130083879081804-0.20051362803279477i], "Freq"=0.0, "ROCOF"=0.0, "ID"=0}, {"Timestamp"=9.433333333333334, "Synx"=[568.0+0.0i, 1.013130277456936-0.20065061735914105i], "Freq"=0.0, "ROCOF"=0.0, "ID"=0}, {"Timestamp"=9.45, "Synx"=[568.0+0.0i, 1.0132687146910482-0.2008004117745078i], "Freq"=0.0, "ROCOF"=0.0, "ID"=0}, {"Timestamp"=9.466666666666667, "Synx"=[568.0+0.0i, 1.0134228065269557-0.20096208726888373i], "Freq"=0.0, "ROCOF"=0.0, "ID"=0}, {"Timestamp"=9.483333333333333, "Synx"=[568.0+0.0i, 1.0135915844590306-0.20113466518863837i], "Freq"=0.0, "ROCOF"=0.0, "ID"=0}, {"Timestamp"=9.5, "Synx"=[568.0+0.0i, 1.0137740095927352-0.20131711799658167i], "Freq"=0.0, "ROCOF"=0.0, "ID"=0}, {"Timestamp"=9.516666666666666, "Synx"=[568.0+0.0i, 1.0139689788840134-0.2015083752378i], "Freq"=0.0, "ROCOF"=0.0, "ID"=0}, {"Timestamp"=9.533333333333333, "Synx"=[568.0+0.0i, 1.0141753324844156-0.20170732967829216i], "Freq"=0.0, "ROCOF"=0.0, "ID"=0}, {"Timestamp"=9.55, "Synx"=[568.0+0.0i, 1.014391861647477-0.2019128435816678i], "Freq"=0.0, "ROCOF"=0.0, "ID"=0}, {"Timestamp"=9.566666666666666, "Synx"=[568.0+0.0i, 1.0146173164979506-0.20212375508799338i], "Freq"=0.0, "ROCOF"=0.0, "ID"=0}, {"Timestamp"=9.583333333333334, "Synx"=[568.0+0.0i, 1.0148504131715899-0.20233888465977073i], "Freq"=0.0, "ROCOF"=0.0, "ID"=0}, {"Timestamp"=9.6, "Synx"=[568.0+0.0i, 1.015089840273925-0.2025570415608225i], "Freq"=0.0, "ROCOF"=0.0, "ID"=0}, {"Timestamp"=9.616666666666667, "Synx"=[568.0+0.0i, 1.0153342650360049-0.20277703033297073i], "Freq"=0.0, "ROCOF"=0.0, "ID"=0}, {"Timestamp"=9.633333333333333, "Synx"=[568.0+0.0i, 1.0155823397338026-0.2029976572349272i], "Freq"=0.0, "ROCOF"=0.0, "ID"=0}, {"Timestamp"=9.65, "Synx"=[568.0+0.0i, 1.015832708794747-0.20321773660935408i], "Freq"=0.0, "ROCOF"=0.0, "ID"=0}, {"Timestamp"=9.666666666666666, "Synx"=[568.0+0.0i, 1.0160840166299678-0.20343609714559968i], "Freq"=0.0, "ROCOF"=0.0, "ID"=0}, {"Timestamp"=9.683333333333334, "Synx"=[568.0+0.0i, 1.016334915820523-0.20365158800555194i], "Freq"=0.0, "ROCOF"=0.0, "ID"=0}, {"Timestamp"=9.7, "Synx"=[568.0+0.0i, 1.0165840750710553-0.20386308478029705i], "Freq"=0.0, "ROCOF"=0.0, "ID"=0}, {"Timestamp"=9.716666666666667, "Synx"=[568.0+0.0i, 1.0168301864324385-0.20406949524737342i], "Freq"=0.0, "ROCOF"=0.0, "ID"=0}, {"Timestamp"=9.733333333333333, "Synx"=[568.0+0.0i, 1.0170719716269168-0.2042697649005633i], "Freq"=0.0, "ROCOF"=0.0, "ID"=0}, {"Timestamp"=9.75, "Synx"=[568.0+0.0i, 1.0173081876979573-0.2044628822248411i], "Freq"=0.0, "ROCOF"=0.0, "ID"=0}, {"Timestamp"=9.766666666666666, "Synx"=[568.0+0.0i, 1.0175376324427896-0.20464788368996814i], "Freq"=0.0, "ROCOF"=0.0, "ID"=0}, {"Timestamp"=9.783333333333333, "Synx"=[568.0+0.0i, 1.0177591500493082-0.20482385843875792i], "Freq"=0.0, "ROCOF"=0.0, "ID"=0}, {"Timestamp"=9.8, "Synx"=[568.0+0.0i, 1.0179716370820475-0.20498995264862666i], "Freq"=0.0, "ROCOF"=0.0, "ID"=0}, {"Timestamp"=9.816666666666666, "Synx"=[568.0+0.0i, 1.0181740486034963-0.20514537354629842i], "Freq"=0.0, "ROCOF"=0.0, "ID"=0}, {"Timestamp"=9.833333333333334, "Synx"=[568.0+0.0i, 1.018365403973238-0.20528939305690688i], "Freq"=0.0, "ROCOF"=0.0, "ID"=0}, {"Timestamp"=9.85, "Synx"=[568.0+0.0i, 1.018544791865278-0.2054213510715208i], "Freq"=0.0, "ROCOF"=0.0, "ID"=0}, {"Timestamp"=9.866666666666667, "Synx"=[568.0+0.0i, 1.0187113742757563-0.20554065831995674i], "Freq"=0.0, "ROCOF"=0.0, "ID"=0}, {"Timestamp"=9.883333333333333, "Synx"=[568.0+0.0i, 1.0188643896266258-0.20564679883739634i], "Freq"=0.0, "ROCOF"=0.0, "ID"=0}, {"Timestamp"=9.9, "Synx"=[568.0+0.0i, 1.0190031553243721-0.2057393320150123i], "Freq"=0.0, "ROCOF"=0.0, "ID"=0}, {"Timestamp"=9.916666666666666, "Synx"=[568.0+0.0i, 1.0191270701753758-0.20581789422765895i], "Freq"=0.0, "ROCOF"=0.0, "ID"=0}, {"Timestamp"=9.933333333333334, "Synx"=[568.0+0.0i, 1.0192356168782655-0.205882200034561i], "Freq"=0.0, "ROCOF"=0.0, "ID"=0}, {"Timestamp"=9.95, "Synx"=[568.0+0.0i, 1.0193283645161266-0.20593204295077844i], "Freq"=0.0, "ROCOF"=0.0, "ID"=0}, {"Timestamp"=9.966666666666667, "Synx"=[568.0+0.0i, 1.0194049707231299-0.20596729578903625i], "Freq"=0.0, "ROCOF"=0.0, "ID"=0}, {"Timestamp"=9.983333333333333, "Synx"=[568.0+0.0i, 1.01946518313326-0.20598791057422627i], "Freq"=0.0, "ROCOF"=0.0, "ID"=0}, {"Timestamp"=10.0, "Synx"=[568.0+0.0i, 1.0195088398631589-0.20599391803560807i], "Freq"=0.0, "ROCOF"=0.0, "ID"=0}] {"Synx" format="%#_4g"}
  out "clEvtReportArray  out":T1 {"Synx" format="%#_4g"}
  in  "btnReadInputData":bool
  in  "btnWriteInputData":bool
  in  "App Plugins":u16(ring)=1 items=["none", "LSE", "Ringdown"]
  in  "btnAppConfigDialog":bool
  in  "btnLoadPlugin":bool
  out "Path":path
  in  "btnRequestINIPath":bool
  in  "btnRemove":bool
  out "Status Log":string
  out "Active Modules (Array)":string[](array[string])
  in  "btnAdd":bool
  in  "btnStop":bool
  in  "Select Module":i32(ring)=-1 caption="Select Module to send Request" items=["All"=-1, "4140002"=4140002, "4140003"=4140003, "4140004"=4140004]
  # "Hidden"
  # "Visible"
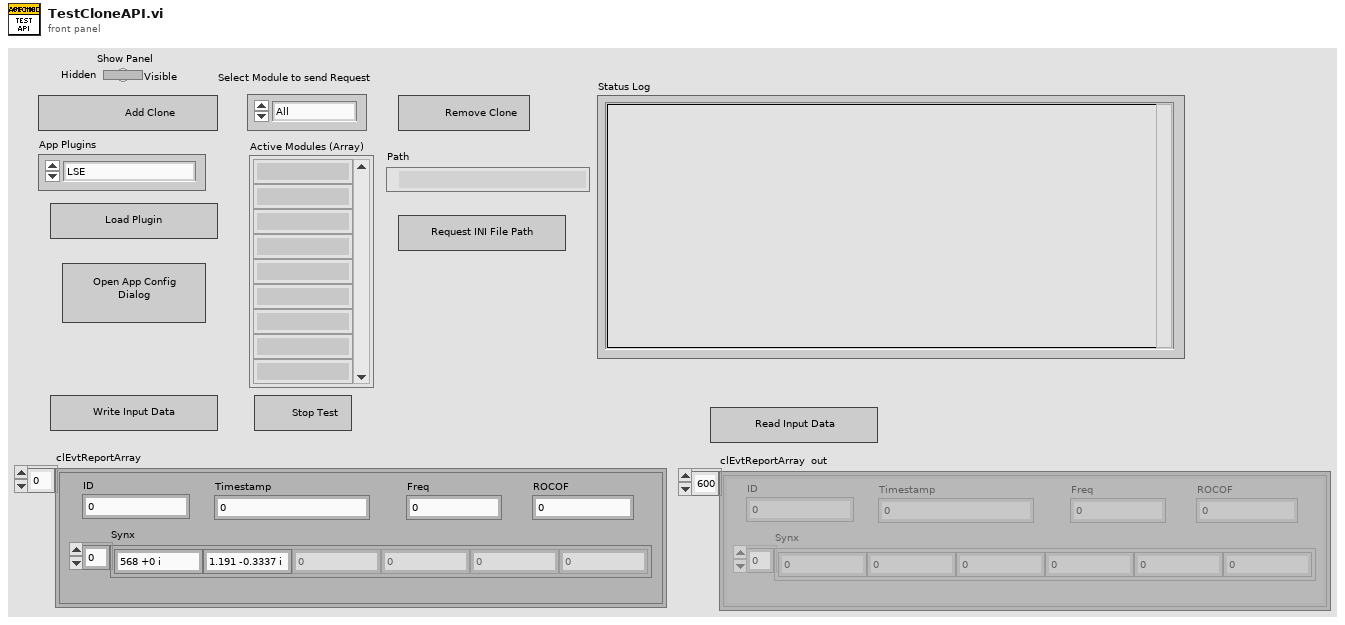
[diagram p1: front panel]
types:
  T1 = typedef "EventPlugins.lvlib/EventPluginBaseClass.lvclass/clEvtReportArray.ctl" = T2[]
  T2 = typedef "EventPlugins.lvlib/EventPluginBaseClass.lvclass/clEvtReport.ctl" = cluster{"Timestamp":dbl, "Synx":cdb[], "Freq":dbl, "ROCOF":dbl, "ID":i16}
  T3 = typedef "AppModule.lvlib/TestInfo.ctl" = cluster{"PluginIniFilePaths":path[]}
  T4 = typedef "AppModule.lvlib/clBroadcastEvents.ctl" = cluster{"DidInit":refnum<user-event>, "StatusUpdate":refnum<user-event>, "ErrorReport":refnum<user-event>, "DidStop":refnum<user-event>, "PathToINI":refnum<user-event>, "InputData":refnum<user-event>, "OutputData":refnum<user-event>, "BcAppInfo":refnum<user-event>, "ConfigData":refnum<user-event>}
  T5 = typedef "AppModule.lvlib/clDidInit.ctl" = cluster{"Init?":bool, "ModuleAdmin":refnum<class "ModuleAdmin.lvclass">}
  T6 = typedef "AppModule.lvlib/clStopArgument.ctl" = cluster{"Exit via Stop Module Req?":bool, "Wait for Module to stop?":bool, "ModuleAdmin":refnum<class "ModuleAdmin.lvclass">}
  T7 = typedef "AppModule.lvlib/clStatUpdate.ctl" = cluster{"Status":string}
  T8 = typedef "AppModule.lvlib/clErrorRpt.ctl" = cluster{"error":errorcluster, "AdditionalInfo":string}
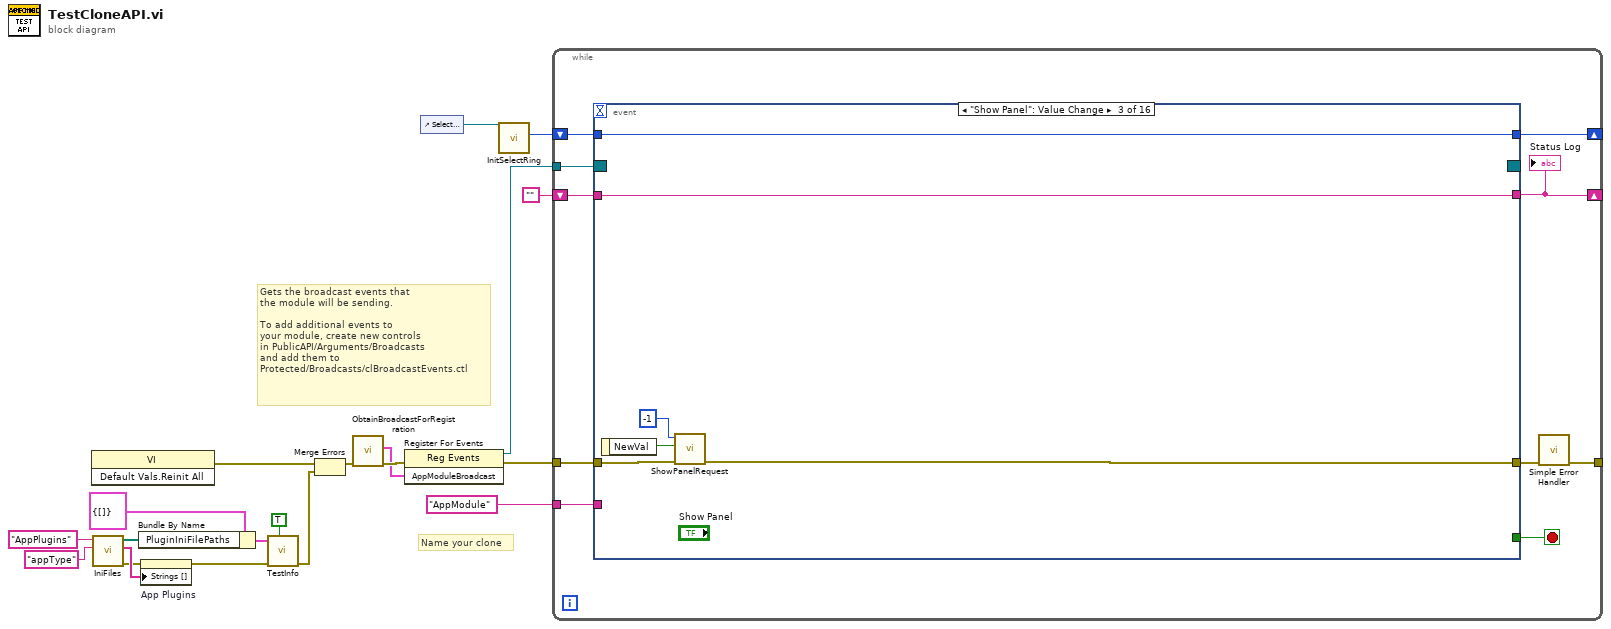
[diagram p0: block diagram]
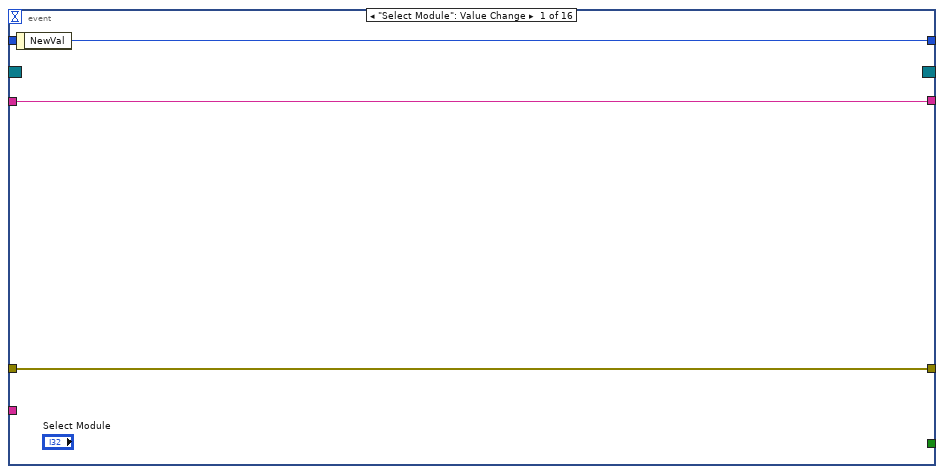
[diagram p2: hidden frame]
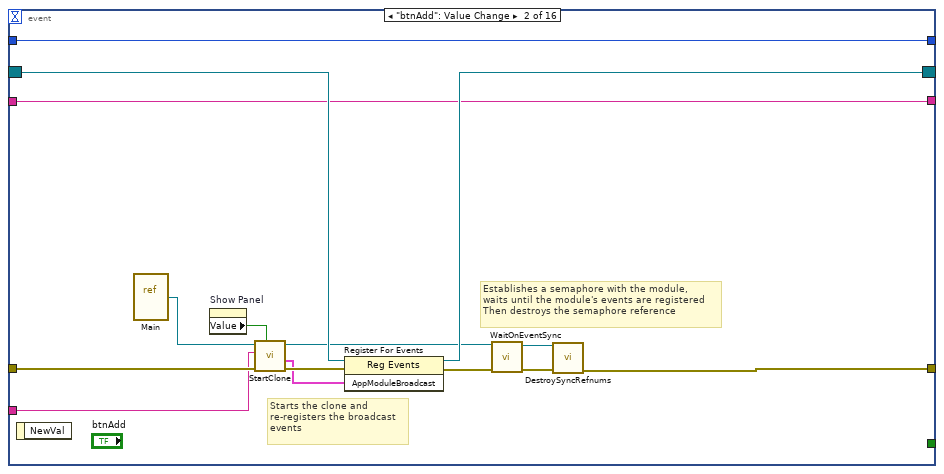
[diagram p3: hidden frame]
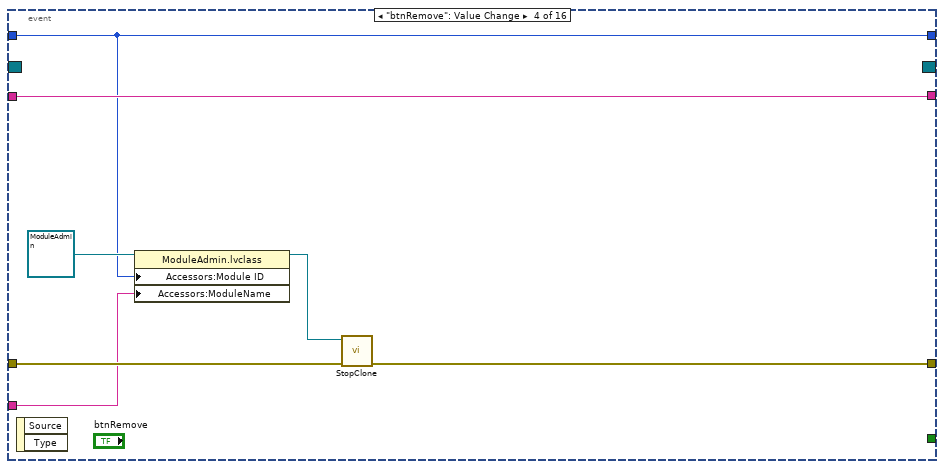
[diagram p4: hidden frame]
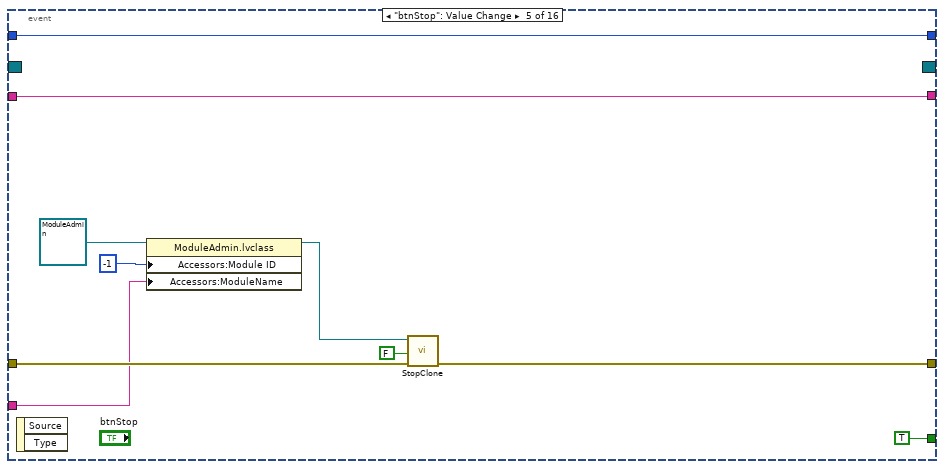
[diagram p5: hidden frame]
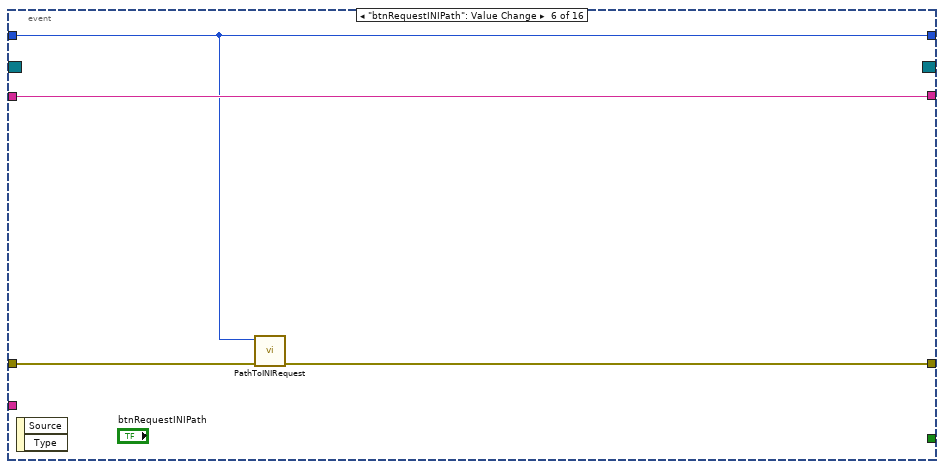
[diagram p6: hidden frame]
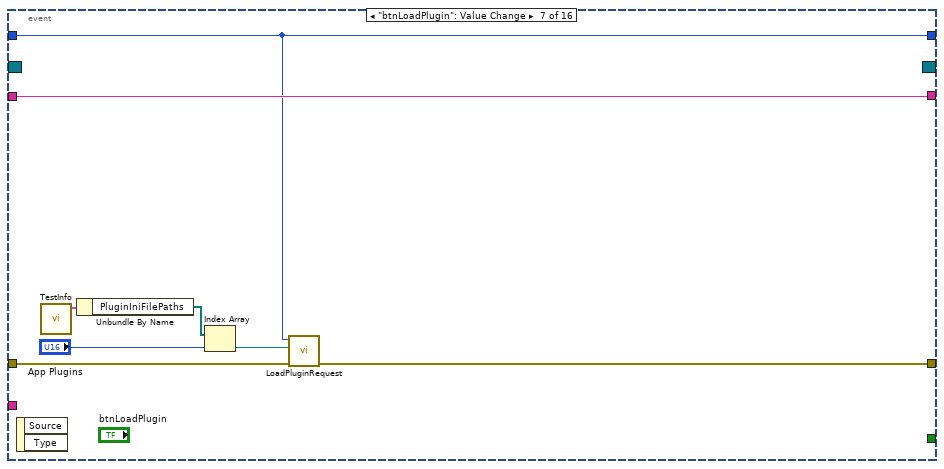
[diagram p7: hidden frame]
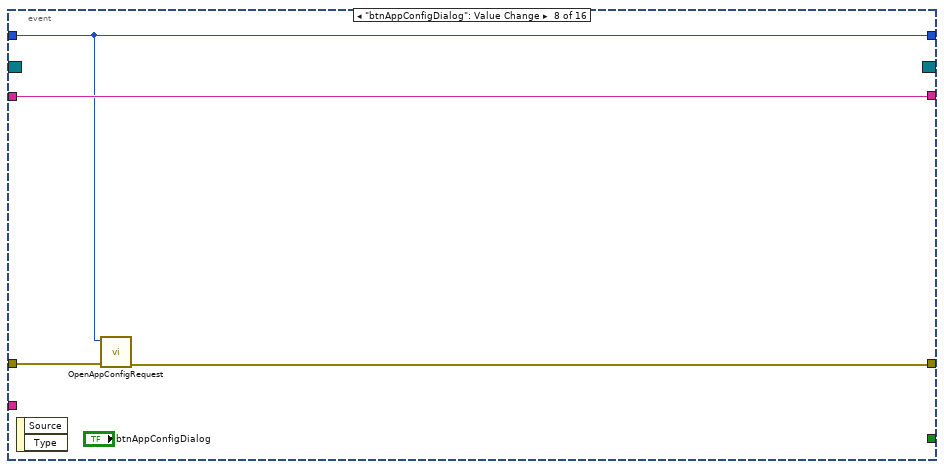
[diagram p8: hidden frame]
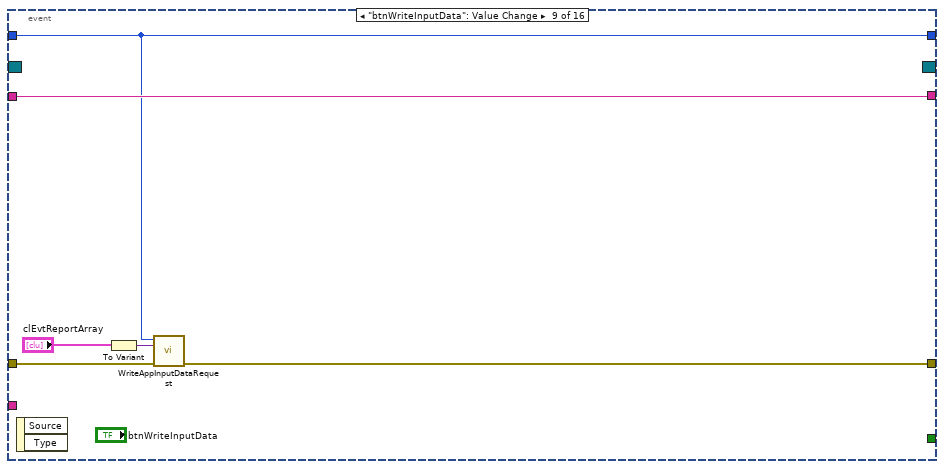
[diagram p9: hidden frame]
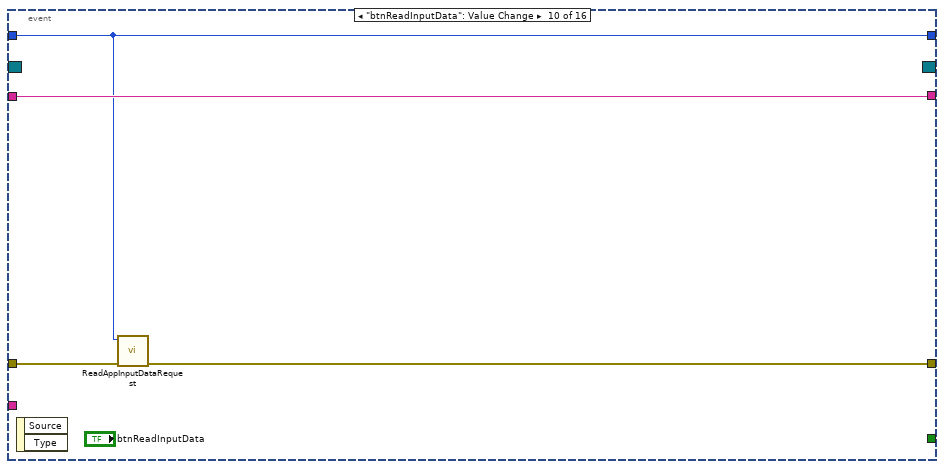
[diagram p10: hidden frame]
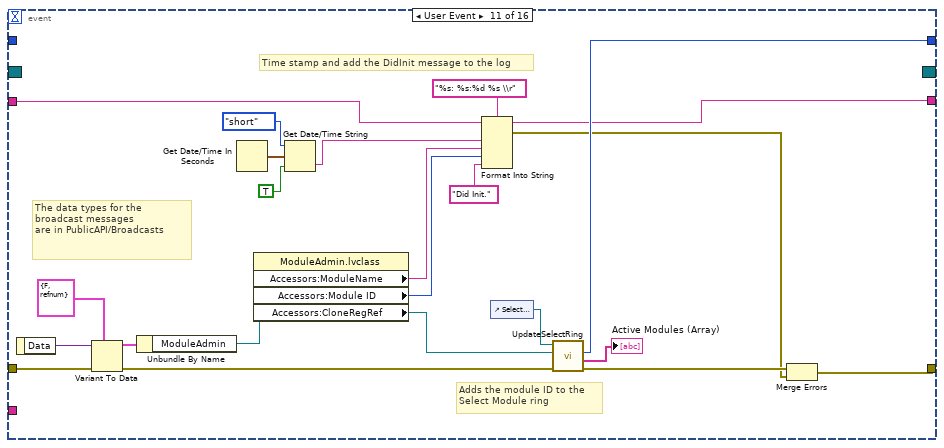
[diagram p11: hidden frame]
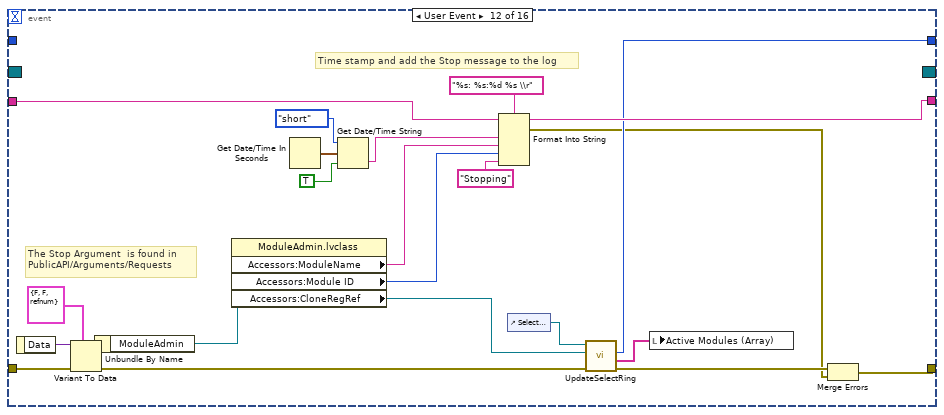
[diagram p12: hidden frame]
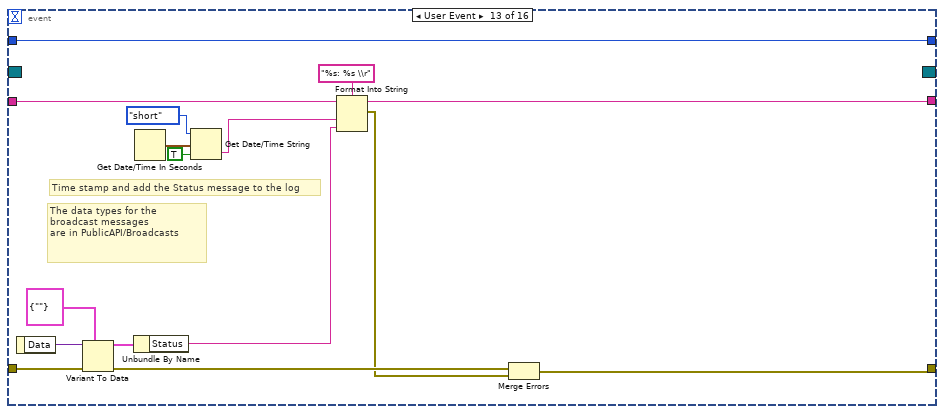
[diagram p13: hidden frame]
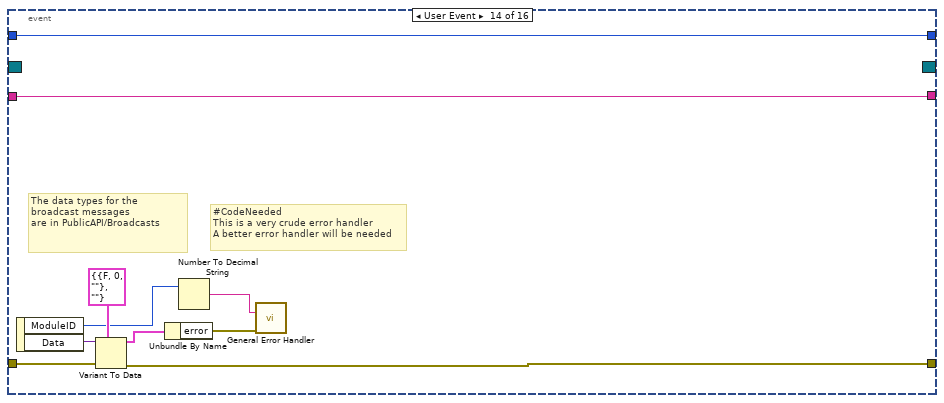
[diagram p14: hidden frame]
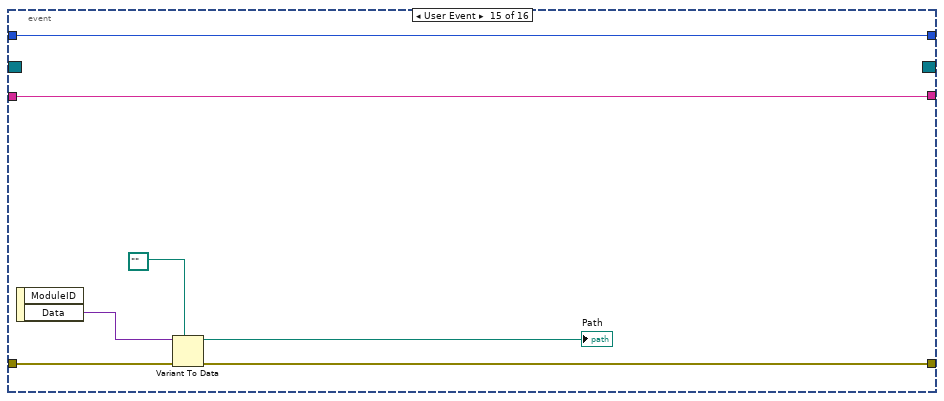
[diagram p15: hidden frame]
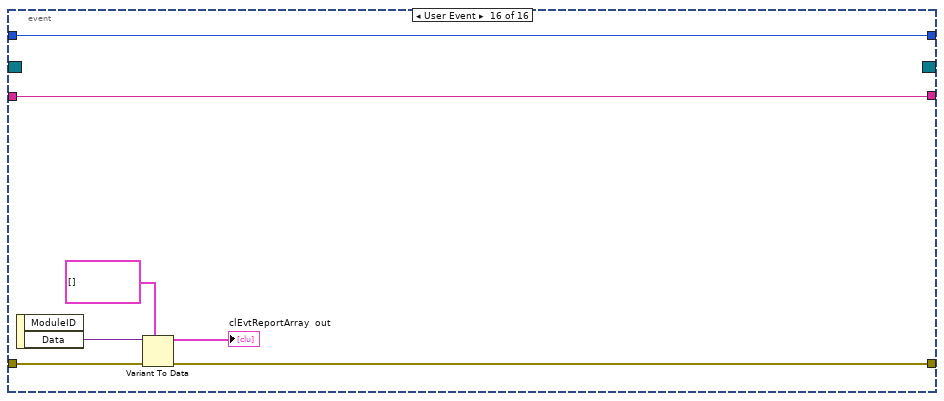
[diagram p16: hidden frame]
diagram:
  # "Name your clone"
  # "Gets the broadcast events that\nthe module will be sending.\n\nTo add additional events to\nyour module, create new controls\nin PublicAPI/Arguments/Broadcasts\nand add them to\nProtected/Broadcasts/clBroadcastEvents.ctl"
  n1 = invoke class="VI" method="Default Vals.Reinit All"() -> (error out=w11:errorcluster)  [unwired: 3 in, 2 out]
  n2 = call "IniFiles.vi"("iniKey"="appType", "name or relative path"="AppPlugins") -> ("error out"=w5:errorcluster, "Types"=w6:string[], "IniFilePaths"=w7:path[])  [unwired: 7 in]
  n3 = Bundle By Name(cluster=T3 {"PluginIniFilePaths"=[]} ("TestInfo"), "PluginIniFilePaths"=w7) -> (w4:T3)
  n4 = property on="App Plugins" class="Ring (strict)"(error in=w5, "Strings []"=w6) -> (error out=w1:errorcluster)  [unwired: 1 in, 1 out]
  n5 = call "TestInfo.vi"("Set (f)"=TRUE, "TestInfo 2"=w4) -> ()  [unwired: 9 in, 1 out]
  n6 = Merge Errors(w11, w1) -> (w2:errorcluster)
  n7 = call "ObtainBroadcastForRegistration.vi"("error in (no error)"=w2) -> ("error out"=w17:errorcluster, "AppModuleBroadcast"=w16:T4)  [unwired: 9 in]
  n8 = register-events(error in=w17, w16) -> (reference out=w14:refnum<event-registration>, error out=w15:errorcluster)  [unwired: 1 in]
  n9 = control-ref of="Select Module"() -> (w19:refnum<vi>)
  n10 = call "InitSelectRing.vi"("Ring Refnum"=w19) -> ("Module Ring Value"=w18:i32)  [unwired: 9 in, 1 out]
  n11 = while {
    shift-right: [w28] -> _
    shift-left: w18 -> [w29]
    tunnel: w15 -> [w26]
    tunnel: w14 -> [w23]
    tunnel: [w24] -> _
    shift-right: [w22] -> _
    shift-left: "" -> [w21]
    tunnel: "AppModule" ("ModuleName") -> [w20]
    stop <- w27 stop-if-true
    n12 = event shown="[2] \"Show Panel\": Value Change" {
      selector: w23 -> [_ w39 _ _ _ _ _ _ _ _ _ _ _ _ _ _]
      dyn-events: [_ w38 _ _ _ _ _ _ _ _ _ _ _ _ _ _] -> _
      timeout: _ -> [_ _ _ _ _ _ _ _ _ _ _ _ _ _ _ _]
      tunnel: w29 -> [_ w47 w49 w56 w70 w73 w80 w84 w88 w94 _ _ w158 w160 w174 w182]
      tunnel: [w32 w47 w49 w56 w70 w73 w80 w84 w88 w94 w114 w129 w158 w160 w174 w182] -> w28
      tunnel: [_ _ _ _ TRUE _ _ _ _ _ _ _ _ _ _ _] -> w27
      tunnel: w26 -> [w30 w46 w53 w59 w68 w72 w81 w85 w92 w95 w119 w138 w155 w167 w170 w180]
      tunnel: [w30 w40 w51 w58 w66 w71 w79 w83 w90 w93 w103 w126 w146 w166 w169 w179] -> w25
      tunnel: [w31 w36 w50 w60 w65 w74 w82 w86 w89 w96 w107 w135 w149 w159 w175 w178] -> w22
      tunnel: w21 -> [w31 w36 w50 w60 w65 w74 w82 w86 w89 w96 w106 w136 w157 w159 w175 w178]
      tunnel: w20 -> [_ w35 _ w55 w62 _ _ _ _ _ _ _ _ _ _ _]
      event "Select Module": Value Change {
        n13 = event-data() -> ("NewVal"=w32:i32)  [unwired: 1 in]
      }
      event "btnAdd": Value Change {
        # "Establishes a semaphore with the module,\nwaits until the module's events are registered\nThen destroys the semaphore reference"
        # "Starts the clone and\nre-registers the broadcast \nevents"
        n14 = event-data() -> ()  [unwired: 1 in, 1 out]
        n15 = vi-ref "Main.vi"() -> (w37:refnum<vi>)
        n16 = property on="Show Panel" class="Bool (strict)"() -> ("Value"=w33:bool)  [unwired: 2 in, 2 out]
        n17 = call "StartClone.vi"("ShowPanel?"=w33, "error in (no error)"=w46, "ModuleName"=w35, "VI Refnum"=w37) -> ("error out"=w45:errorcluster, "clBroadcastEvents"=w41:T4, "ModuleAdmin"=w34:refnum<class "ModuleAdmin.lvclass">)  [unwired: 5 in]
        n18 = register-events(reference=w39, error in=w45, w41) -> (reference out=w38:refnum<event-registration>, error out=w44:errorcluster)
        n19 = call <userlib>:"WaitOnEventSync.vi"("error in (no error)"=w44, "ModuleAdmin"=w34) -> ("error out"=w43:errorcluster, "ModuleAdmin"=w42:refnum<class "ModuleAdmin.lvclass">)  [unwired: 8 in]
        n20 = call <userlib>:"DestroySyncRefnums.vi"("error in (no error)"=w43, "ModuleAdmin"=w42) -> ("error out"=w40:errorcluster)  [unwired: 9 in]
      }
      event "Show Panel": Value Change {
        n21 = event-data() -> ("NewVal"=w52:bool)  [unwired: 1 in]
        n22 = call "ShowPanelRequest.vi"("error in (no error)"=w53, "ShowPanel"=w52, "ModuleID"=-1) -> ("error out"=w51:errorcluster)  [unwired: 8 in]
      }
      event "btnRemove": Value Change {
        n23 = event-data() -> ()  [unwired: 1 in, 2 out]
        n24 = property class="ModuleAdmin.lvclass"(reference=refnum<class "ModuleAdmin.lvclass"> refnum ("NistModuleAdmin.lvlib:NistModuleAdmin.lvclass"), "Accessors:Module ID"=w56, "Accessors:ModuleName"=w55) -> (reference out=w54:refnum<class "ModuleAdmin.lvclass">)  [unwired: 1 in, 1 out]
        n25 = call "StopClone.vi"("error in (no error)"=w59, "ModuleAdmin"=w54) -> ("error out"=w58:errorcluster)  [unwired: 9 in]
      }
      event "btnStop": Value Change {
        n26 = event-data() -> ()  [unwired: 1 in, 2 out]
        n27 = property class="ModuleAdmin.lvclass"(reference=refnum<class "ModuleAdmin.lvclass"> refnum ("NistModuleAdmin.lvlib:NistModuleAdmin.lvclass"), "Accessors:Module ID"=-1 ("Module ID"), "Accessors:ModuleName"=w62) -> (reference out=w61:refnum<class "ModuleAdmin.lvclass">)  [unwired: 1 in, 1 out]
        n28 = call "StopClone.vi"("error in (no error)"=w68, "Wait for Module to stop?"=FALSE, "ModuleAdmin"=w61) -> ("error out"=w66:errorcluster)  [unwired: 8 in]
      }
      event "btnRequestINIPath": Value Change {
        n29 = event-data() -> ()  [unwired: 1 in, 2 out]
        n30 = call "PathToINIRequest.vi"("error in (no error)"=w72, "ModuleID"=w73) -> ("error out"=w71:errorcluster)  [unwired: 9 in]
      }
      event "btnLoadPlugin": Value Change {
        n31 = event-data() -> ()  [unwired: 1 in, 2 out]
        n32 = call "TestInfo.vi"() -> ("TestInfo"=w78:T3)  [unwired: 11 in]
        n33 = Unbundle By Name(w78) -> ("PluginIniFilePaths"=w76:path[])
        n34 = Index Array(array=w76, index="App Plugins") -> (element=w75:path)
        n35 = call "LoadPluginRequest.vi"("error in (no error)"=w81, "PathToPluginINI"=w75, "ModuleID"=w80) -> ("error out"=w79:errorcluster)  [unwired: 8 in]
      }
      event "btnAppConfigDialog": Value Change {
        n36 = event-data() -> ()  [unwired: 1 in, 2 out]
        n37 = call "OpenAppConfigRequest.vi"("error in (no error)"=w85, "ModuleID"=w84) -> ("error out"=w83:errorcluster)  [unwired: 9 in]
      }
      event "btnWriteInputData": Value Change {
        n38 = event-data() -> ()  [unwired: 1 in, 2 out]
        n39 = To Variant(anything="clEvtReportArray") -> (Variant=w91:variant)
        n40 = call "WriteAppInputDataRequest.vi"("error in (no error)"=w92, "InputData"=w91, "ModuleID"=w88) -> ("error out"=w90:errorcluster)  [unwired: 8 in]
      }
      event "btnReadInputData": Value Change {
        n41 = event-data() -> ()  [unwired: 1 in, 2 out]
        n42 = call "ReadAppInputDataRequest.vi"("error in (no error)"=w95, "ModuleID"=w94) -> ("error out"=w93:errorcluster)  [unwired: 9 in]
      }
      event User Event {
        # "Adds the module ID to the \nSelect Module ring"
        # "Time stamp and add the DidInit message to the log"
        # "The data types for the broadcast messages\nare in PublicAPI/Broadcasts"
        n43 = event-data() -> ("Data"=w118:variant)  [unwired: 1 in]
        n44 = Variant To Data(error in=w119, type=T5 {"Init?"=FALSE, "ModuleAdmin"=refnum} ("clDidInit"), Variant=w118) -> (data=w111:T5, error out=w116:errorcluster)
        n45 = Unbundle By Name(w111) -> ("ModuleAdmin"=w101:refnum<class "ModuleAdmin.lvclass">)
        n46 = Get Date/Time In Seconds() -> (seconds since 1Jan1904=w109:timestamp)
        n47 = property class="ModuleAdmin.lvclass"(reference=w101) -> ("Accessors:ModuleName"=w99:string, "Accessors:Module ID"=w98:i32, "Accessors:CloneRegRef"=w97:refnum<data-value>)  [unwired: 1 in, 2 out]
        n48 = Get Date/Time String(date format (0)=enum16{"short", "long", "abbreviated"}."short", seconds (now)=w109, want seconds? (F)=TRUE) -> (time string=w112:string)  [unwired: 1 out]
        n49 = Format Into String(format string="%s: %s:%d %s \\r", initial string=w106, w112, w99, w98, "Did Init.") -> (resulting string=w107:string, error out=w104:errorcluster)  [unwired: 1 in]
        n50 = control-ref of="Select Module"() -> (w115:refnum<vi>)
        n51 = call "UpdateSelectRing.vi"("error in (no error)"=w116, "CloneRegRef"=w97, "Ring Refnum"=w115) -> ("error out"=w105:errorcluster, "ActiveModules"=→"Active Modules (Array)":string[], "Module Ring Value"=w114:i32)  [unwired: 6 in]
        n52 = Merge Errors(w105, w104) -> (w103:errorcluster)
      }
      event User Event {
        # "Time stamp and add the Stop message to the log"
        # "The Stop Argument  is found in\nPublicAPI/Arguments/Requests"
        n53 = event-data() -> ("Data"=w137:variant)  [unwired: 1 in]
        n54 = Variant To Data(error in=w138, type=T6 {"Exit via Stop Module Req?"=FALSE, "Wait for Module to stop?"=FALSE, "ModuleAdmin"=refnum} ("Stop Argument"), Variant=w137) -> (data=w133:T6, error out=w132:errorcluster)
        n55 = Unbundle By Name(w133) -> ("ModuleAdmin"=w124:refnum<class "ModuleAdmin.lvclass">)
        n56 = property class="ModuleAdmin.lvclass"(reference=w124) -> ("Accessors:ModuleName"=w122:string, "Accessors:Module ID"=w121:i32, "Accessors:CloneRegRef"=w120:refnum<data-value>)  [unwired: 1 in, 2 out]
        n57 = Get Date/Time In Seconds() -> (seconds since 1Jan1904=w140:timestamp)
        n58 = Get Date/Time String(date format (0)=enum16{"short", "long", "abbreviated"}."short", seconds (now)=w140, want seconds? (F)=TRUE) -> (time string=w142:string)  [unwired: 1 out]
        n59 = Format Into String(format string="%s: %s:%d %s \\r", initial string=w136, w142, w122, w121, "Stopping") -> (resulting string=w135:string, error out=w127:errorcluster)  [unwired: 1 in]
        n60 = control-ref of="Select Module"() -> (w131:refnum<vi>)
        n61 = call "UpdateSelectRing.vi"("error in (no error)"=w132, "CloneRegRef"=w120, "Ring Refnum"=w131) -> ("error out"=w128:errorcluster, "ActiveModules"=w130:string[], "Module Ring Value"=w129:i32)  [unwired: 6 in]
        n62 = local write "Active Modules (Array)"(w130) -> ()
        n63 = Merge Errors(w128, w127) -> (w126:errorcluster)
      }
      event User Event {
        # "Time stamp and add the Status message to the log"
        # "The data types for the broadcast messages\nare in PublicAPI/Broadcasts"
        n64 = event-data() -> ("Data"=w154:variant)  [unwired: 1 in]
        n65 = Variant To Data(error in=w155, type=T7 {"Status"=""} ("clStatUpdate"), Variant=w154) -> (data=w152:T7, error out=w148:errorcluster)
        n66 = Unbundle By Name(w152) -> ("Status"=w150:string)
        n67 = Get Date/Time In Seconds() -> (seconds since 1Jan1904=w151:timestamp)
        n68 = Get Date/Time String(date format (0)=enum16{"short", "long", "abbreviated"}."short", seconds (now)=w151, want seconds? (F)=TRUE) -> (time string=w143:string)  [unwired: 1 out]
        n69 = Format Into String(format string="%s: %s \\r", initial string=w157, w143, w150) -> (resulting string=w149:string, error out=w147:errorcluster)  [unwired: 1 in]
        n70 = Merge Errors(w148, w147) -> (w146:errorcluster)
      }
      event User Event {
        # "#CodeNeeded\nThis is a very crude error handler\nA better error handler will be needed"
        # "The data types for the broadcast messages\nare in PublicAPI/Broadcasts"
        n71 = event-data() -> ("ModuleID"=w163:i32, "Data"=w168:variant)  [unwired: 1 in]
        n72 = Variant To Data(error in=w167, type=T8 {"error"={"status"=FALSE, "code"=0, "source"=""}, "AdditionalInfo"=""} ("Cluster"), Variant=w168) -> (data=w164:T8, error out=w166:errorcluster)
        n73 = Unbundle By Name(w164) -> ("error"=w162:errorcluster)
        n74 = Number To Decimal String(number=w163) -> (decimal integer string=w161:string)  [unwired: 1 in]
        n75 = call <vilib>:"General Error Handler.vi"("[error source] (\" \")"=w161, "error in (no error)"=w162) -> ()  [unwired: 9 in, 5 out]
      }
      event User Event {
        n76 = event-data() -> ("Data"=w172:variant)  [unwired: 1 in, 1 out]
        n77 = Variant To Data(error in=w170, type=path "" ("Path"), Variant=w172) -> (data=→"Path":path, error out=w169:errorcluster)
      }
      event User Event {
        n78 = event-data() -> ("Data"=w181:variant)  [unwired: 1 in, 1 out]
        n79 = Variant To Data(error in=w180, type=T1 [] ("clEvtReportArray"), Variant=w181) -> (data=→"clEvtReportArray  out":T1, error out=w179:errorcluster)
      }
    }
    "Status Log" <- w22
    n80 = call <vilib>:"Simple Error Handler.vi"("error in (no error)"=w25) -> ("error out"=w24:errorcluster)  [unwired: 4 in, 4 out]
  }
